vi "BRig_RT_start_v1,05__PortC.vi"() -> ()   [LabVIEW 2014]
uses:
  myRIO_BRig_RT__Case_Exp_stateList.ctl
  myRIO_BRig_RT__Case_NonExp_stateList.ctl
  <vilib>/WebDAVClient/Advanced/SessionHandle.ctl
  <vilib>/Platform/TimedLoop/XDataNode/timing_clust.ctl
  <vilib>/Platform/TimedLoop/XDataNode/nitl_modes.ctl
  <vilib>/Platform/TimedLoop/XDataNode/wakeup.ctl
  <vilib>/myRIO/Common/Instrument Driver Framework/myRIO v1.0/UART/vis/myRIO v1.0 Close UART.vi
  <vilib>/FPGAPlugInAG/myRIO-1900/niLvFpga_Open_myRIO-1900.vi
  <vilib>/rvi/interface/common/dynamic/niFpgaDynamicAddResources.vi
  <vilib>/Utility/error.llb/Error Cluster From Error Code.vi
  <vilib>/rvi/errors/niLvFpgaAdjustHostInterfaceError.vi
  <vilib>/Utility/file.llb/Read From Spreadsheet File (I64).vi
  <vilib>/Utility/file.llb/Write To Spreadsheet File (DBL).vi
  <vilib>/FPGAPlugInAG/Dynamic/niLvFpga_Close_Dynamic.vi
  <vilib>/myRIO/Common/Instrument Driver Framework/Utilities/vis/FPGA Ref Manager.vi
  <vilib>/myRIO/Common/Instrument Driver Framework/myRIO v1.0/myRIO v1.0 Reset FPGA.vi
  <vilib>/myRIO/Common/Instrument Driver Framework/myRIO v1.0/IRQ/vis/myRIO v1.0 IRQ Info FGV.vi
  <vilib>/myRIO/Common/Instrument Driver Framework/myRIO v1.0/IRQ/vis/myRIO v1.0 Timer IRQ Info FGV.vi
  <vilib>/myRIO/Common/Instrument Driver Framework/myRIO v1.0/IRQ/vis/myRIO v1.0 ISR Agent.vi
  <vilib>/rvi/interface/nirviOpenFPGA/nirviOpenFPGA.xnode
  BRig_FPGA_v3,91__PortC__build.lvbitx
  BRig_FPGA_v3,91__PortC.vi
  <vilib>/rvi/interface/nirviReadWriteControl/nirviReadWriteControl.xnode
  <vilib>/Platform/TimedLoop/XDataNode/XDataNode.xnode
  <vilib>/rvi/interface/nirviCloseFPGA/nirviCloseFPGA.xnode
  <vilib>/Platform/TimedLoop/XDataNode/XDNodeRunTimeDep.lvlib
  <vilib>/rvi/interface/Simulation/niFpgaSimulationCallBeginRW.vi
  <vilib>/myRIO/Instrument Drivers/Utilities/Utilities.lvlib
  NiFpgaLv.dll
  <vilib>/WebDAVClient/NI_WebDAV.lvlib
panel:
  out "FreeReward_c_R":u16
  out "FreeReward_c_L":u16
  in  "Laser2_LED":bool
  in  "Laser1_LED":bool
  in  "lick_Rising(F)_or_Falling(T)":bool
  out "T_ExpRun_min":dbl
  out "stop_TimedLoop":bool
  out "BTPR_avg_R":dbl
  out "T2R_avg_R":dbl
  out "BTPR_avg_L":dbl
  out "T2R_avg_L":dbl
  out "BTPR_block":u16
  out "T2R_block":u16
  in  "comm_WebDAV_connect":bool
  in  "I_sendData":bool
  in  "comm_TCP_connect":bool
  out "nRewards_total":u16 caption="# Rewards in Current Block"
  out "BUR_target":u16 caption="Target Trials Per Block"
  in  "input_Threshold_reset":bool
  out "nTrial":u16
  out "allReward_R":bool
  out "allReward_L":bool
  out "Threshold":bool
  out "tLoop":dbl format="%#_2g"
  out "L_Power_l2":dbl
  out "comm_TCP":bool
  in  "get_countPerMS":bool
  out "SolenoidReward":bool
  out "L_Power_l1":dbl caption="LaserPower"
  in  "Recording":bool
  out "FPGA_count2ms":dbl=159.0
  out "error out":errorcluster
  out "cSpout":enum16{"Left", "Right"}(ring) caption="Left or Right Spout"
  out "A4":u32 caption="LickCounter_Right"
  out "A2":u32 caption="LickCounter_Left"
  out "nRewards_Right":u16 caption="# Rewards Total (Right)"
  out "nRewards_Left":u16 caption="# Rewards Total (Left)"
  out "nRewards_cur":u16 caption="# Rewards in Current Block"
  out "TpB_target":u16 caption="Target Trials Per Block"
  out "cState_NonExp":T1 caption="WarmUp State"
  out "iBlock":u16 caption="Current Block"
  out "cState":T2 caption="Experimental State"
  out "iTrial":u16 caption="Current Trial"
  in  "Data Set Prefix":string="Exp1_TM2"
  out "comm_WebDAV":bool
  in  "Host Password":string="sabalab"
  in  "Host UserName":string="Test2"
  in  "STOP_abort":bool caption="Stop LabView\n(Stops myRio and FPGA)"
  in  "STOP_endBlock":bool caption="Stop Experiment\n@ End of Block"
  in  "STOP_endTrial":bool caption="Stop Experiment\n@ End of Trial"
  in  "START":bool caption="Start Experiment"
  # "Experimental Run"
  # "Recording Rig"
  # "FPGA Conversion\n[counts per ms]"
  # "RealTime Cycle\nShould be <5ms"
  # "STOP experiment at"
  # "Exp Run Time"
  # "Reset"
  # "min"
  # "Communication with Host"
  # "Test AnalogInput Plotting"
  # "Lick Counter"
  # "Give Water?\n(Reward)"
  # "Experimental State"
  # "Left/Right"
  # "AI0               AI1"
  # "Left           Right"
  # "Direction\n(NonSpecific Licking)"
  # "Block Target"
  # "# Blocks"
  # "L          R"
  # "# Trials"
  # "# Rewards"
  # "Bad Trials\nPost Reward"
  # "Trials 2 Reward"
  # "Block"
  # "# Trials"
  # "# Rewards"
  # "Current\nBlock"
  # "WarmUp State"
  # "avg L"
  # "Total"
  # "# Rewards"
  # "# Trials"
  # "avg R"
  # "Laser Power [V]"
  # "Left           Right"
  # "FreeRewards"
  # "Laser1"
  # "Laser2"
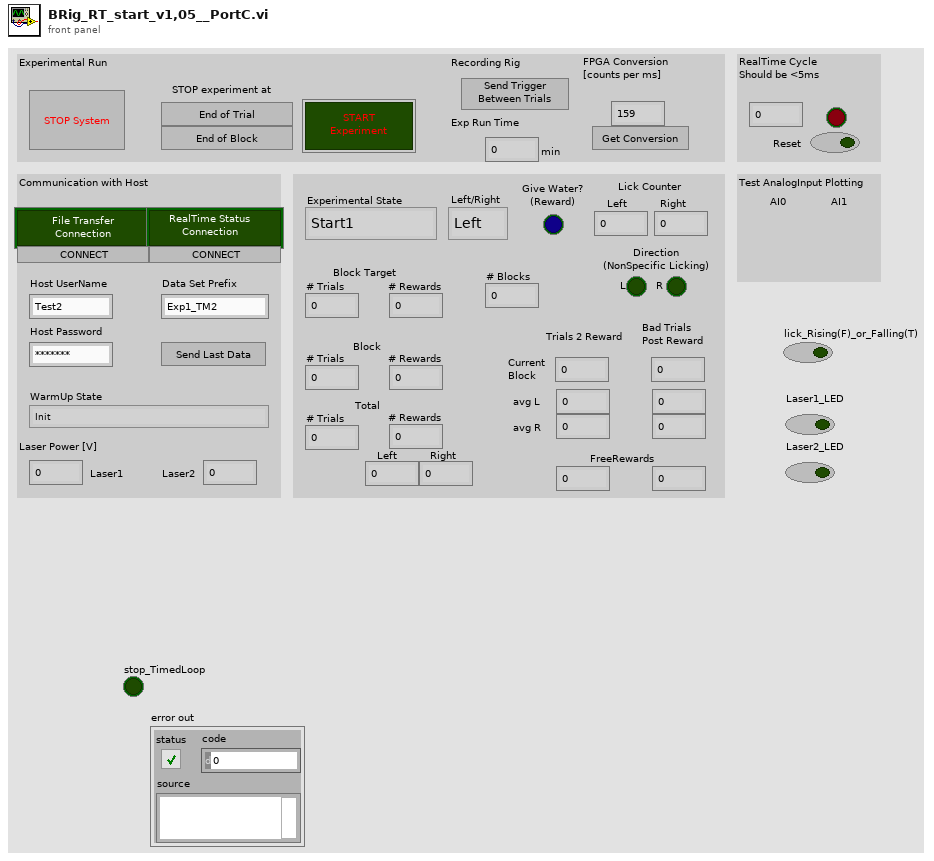
[diagram p1: front panel]
types:
  T1 = typedef "myRIO_BRig_RT__Case_NonExp_stateList.ctl" = enum16{"Init", "UploadSettings_pre", "UploadSettings_Read_dataExp", "UploadSettings_dataExp_1", "UploadSettings_dataExp_2", "UploadSettings_Read_dataLC", "UploadSettings_dataLC_1", "UploadSettings_dataLC_2", "UploadSettings_dataLC_3", "UploadSettings_dataLC_4", "UploadSettings_Read_dataMTrig", "UploadSettings_dataMTrig_1", "UploadSettings_post", "Idle_pre", "IdleEmpty", "IdleEmpty2", "IdleEmpty3", "IdleEmpty4", "Idle", "Idle_2", "Idle_3", "Idle_4", "Idle_5", "Idle_6", "Idle_post", "Cue_pre__pre", "Cue_pre", "Cue", "Cue_LED", "Cue_post", "RewardCalibration_pre", "RewardCalibration", "DispenseWater_pre__pre", "DispenseWater_pre", "DispenseWater", "DispenseWater_post", "TestConnection", "SendData", "Get_FPGA_count_per_ms", "End", "commTCP_connect"}
  T2 = typedef "myRIO_BRig_RT__Case_Exp_stateList.ctl" = enum16{"Start1", "Start2", "Start3", "saveSettings1", "saveSettings2", "saveSettings3", "saveSettings4", "saveSettings_LC_ENL_l1", "saveSettings_LC_ENL_l2", "saveSettings_LC_Cue_l1", "saveSettings_LC_Cue_l2", "saveSettings6_LC_l1_Other", "SaveSettings6_LC_l2_Other", "setSettings_Audio", "setSettings_Laser", "initBlock_pre", "initBlock", "initBlock2", "initBlock_post", "initTrial_pre", "initTrial", "initTrial2", "initTrial3", "initTrial4", "initTrial_LC_ENL1", "initTrial_LC_Cue1", "initTrial_LC_Cue1_2", "initTrial_LC_Sel", "initTrial_post", "ENL1_pre", "ENL1", "ENL1_post", "ENL1Penalty_pre", "ENL1Penalty", "ENL2_pre", "ENL2", "ENL2Penalty_pre", "ENL2Penalty", "Cue1_pre", "Cue1", "Cue1_post", "Cue1Penalty_pre", "Cue1Penalty", "Cue2_pre", "Cue2", "Cue2Penalty_pre", "Cue2Penalty", "Selection_pre", "Selection", "Select_post", "SelectReward_pre", "SelectReward", "SelectRewardPost_pre", "SelectRewardPost", "SelectWrong_pre", "SelectWrong", "SelectWrong_post", "SelectTimeout_pre", "SelectTimeout", "SelectTimeout_post", "endTrial_pre", "endTrial1", "endTrial2", "endTrial3", "endTrial_post", "endBlock_pre", "endBlock", "endBlock_post", "endExp", "commConnect", "commUpload_pre", "commUpload_dataBlock", "commUpload_dataCurrent", "commUpload_dataExp", "commUpload_dataLC", "commUpload_dataTrial", "commUpload_post", "saveData_pre", "saveData_dataBlock", "saveData_dataCurrent", "saveData_dataExp", "saveData_dataLC", "saveData_dataTrial", "saveData_post", "empty_endBlock1", "empty_endBlock2", "empty_endTrial1", "empty_endTrial2", "empty_endTrial3", "empty_endTrial4", "empty_endTrial5", "dummyState", "dummyState_endBlock", "FreeReward_pre", "FreeReward", "FreeRewardPost_pre", "FreeRewardPost"}
  T3 = enum8{"Enabled", "Disabled", "Disabled and Grayed Out"}
  T4 = typedef "NI_WebDAV.lvlib/SessionHandle.ctl" = refnum<k1>
  T5 = typedef "XDNodeRunTimeDep.lvlib/timing_clust.ctl" = cluster{"Expected End [f-1]":u64, "Actual End [f-1]":u64, "Finished Late? [f-1]":bool, "Expected End [i-1]":u64, "Actual End [i-1]":u64, "Finished Late? [i-1]":bool, "Expected Start [i]":u64, "Actual Start [i]":u64, "Expected Start [f]":u64, "Actual Start [f]":u64, "Source Name":string, "Structure Name":string, "Period":i64, "Deadline":i64, "Offset":i64, "Start":i64, "Priority":i32, "Timeout":i32, "Mode":T6, "Wakeup Reason":T7, "Error":errorcluster, "Source Type":string, "Secondary Source Type":string, "Global End Time":u64, "Global Start Time":u64, "Frame Duration":u64, "Iteration Duration":u64, "Assigned CPU":i32, "I/O Scan Engine Mode":u32}
  T6 = typedef "XDNodeRunTimeDep.lvlib/nitl_modes.ctl" = enum32{"No Change", "Process missed periods, maintain original phase", "Discard missed periods, maintain original phase", "Process missed periods, ignore original phase", "Discard missed periods, ignore original phase"}
  T7 = typedef "XDNodeRunTimeDep.lvlib/wakeup.ctl" = enum32{"Normal", "Aborted", "Asynchronous wakeup", "Timing source error", "Timed loop error", "Timeout"}
  T8 = cluster{"read mode":enum16{"polling", "blocking"}, "write mode":enum16{"polling", "blocking"}}
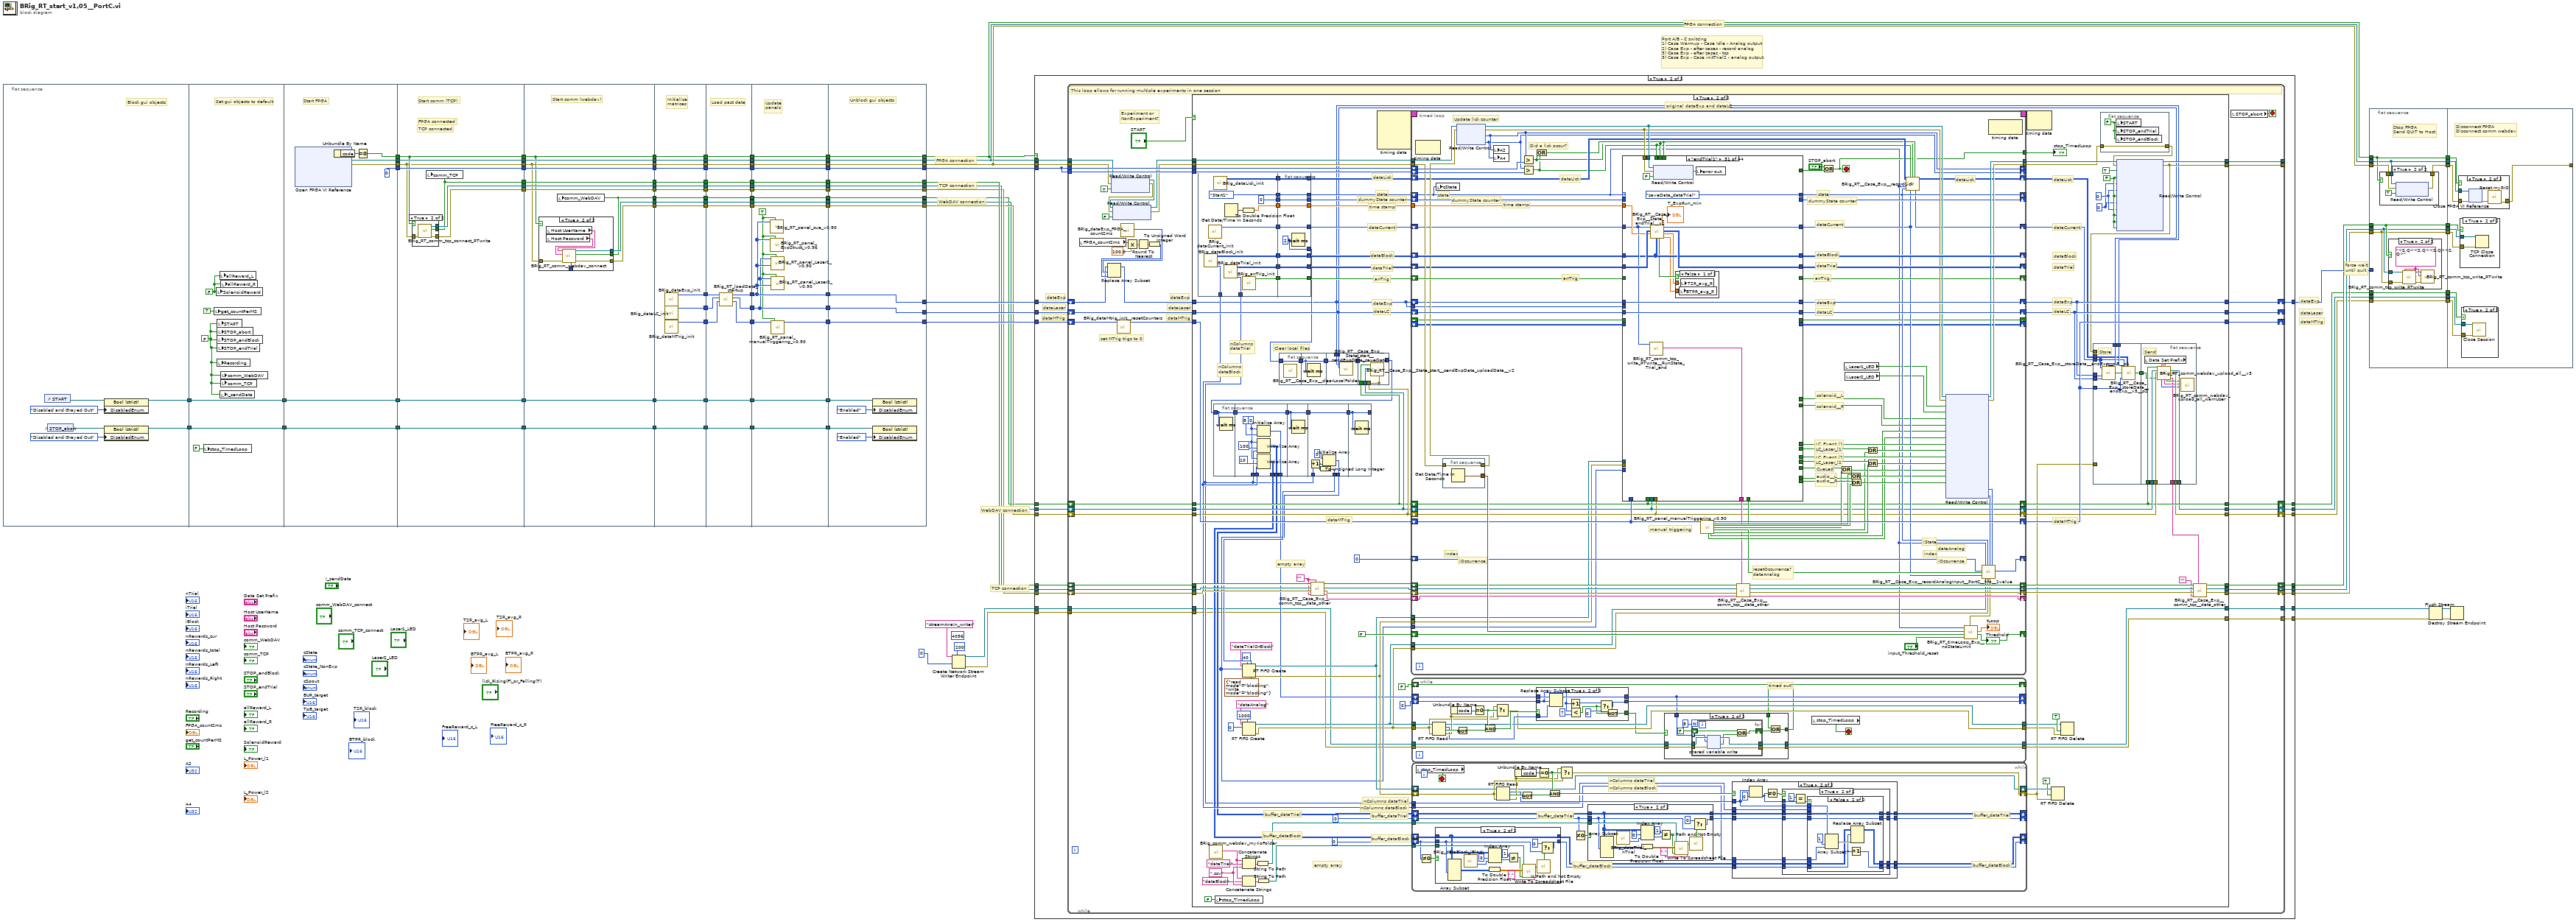
[diagram p0: block diagram]
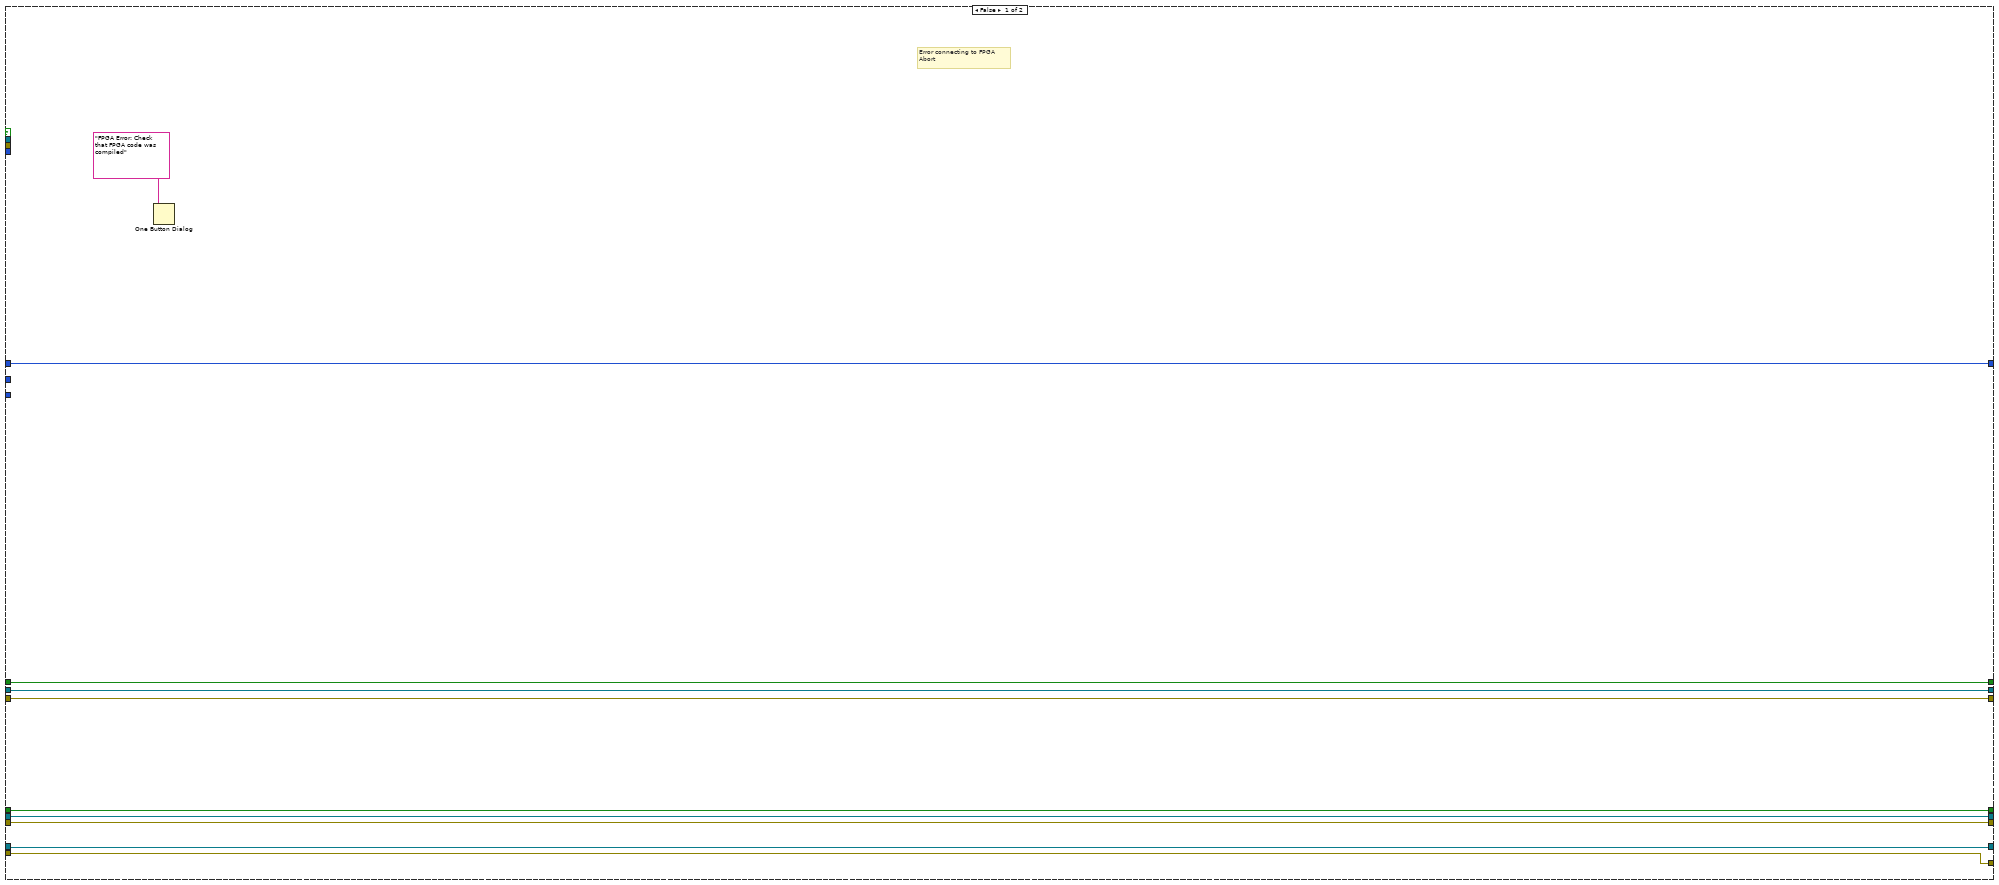
[diagram p2: hidden frame]
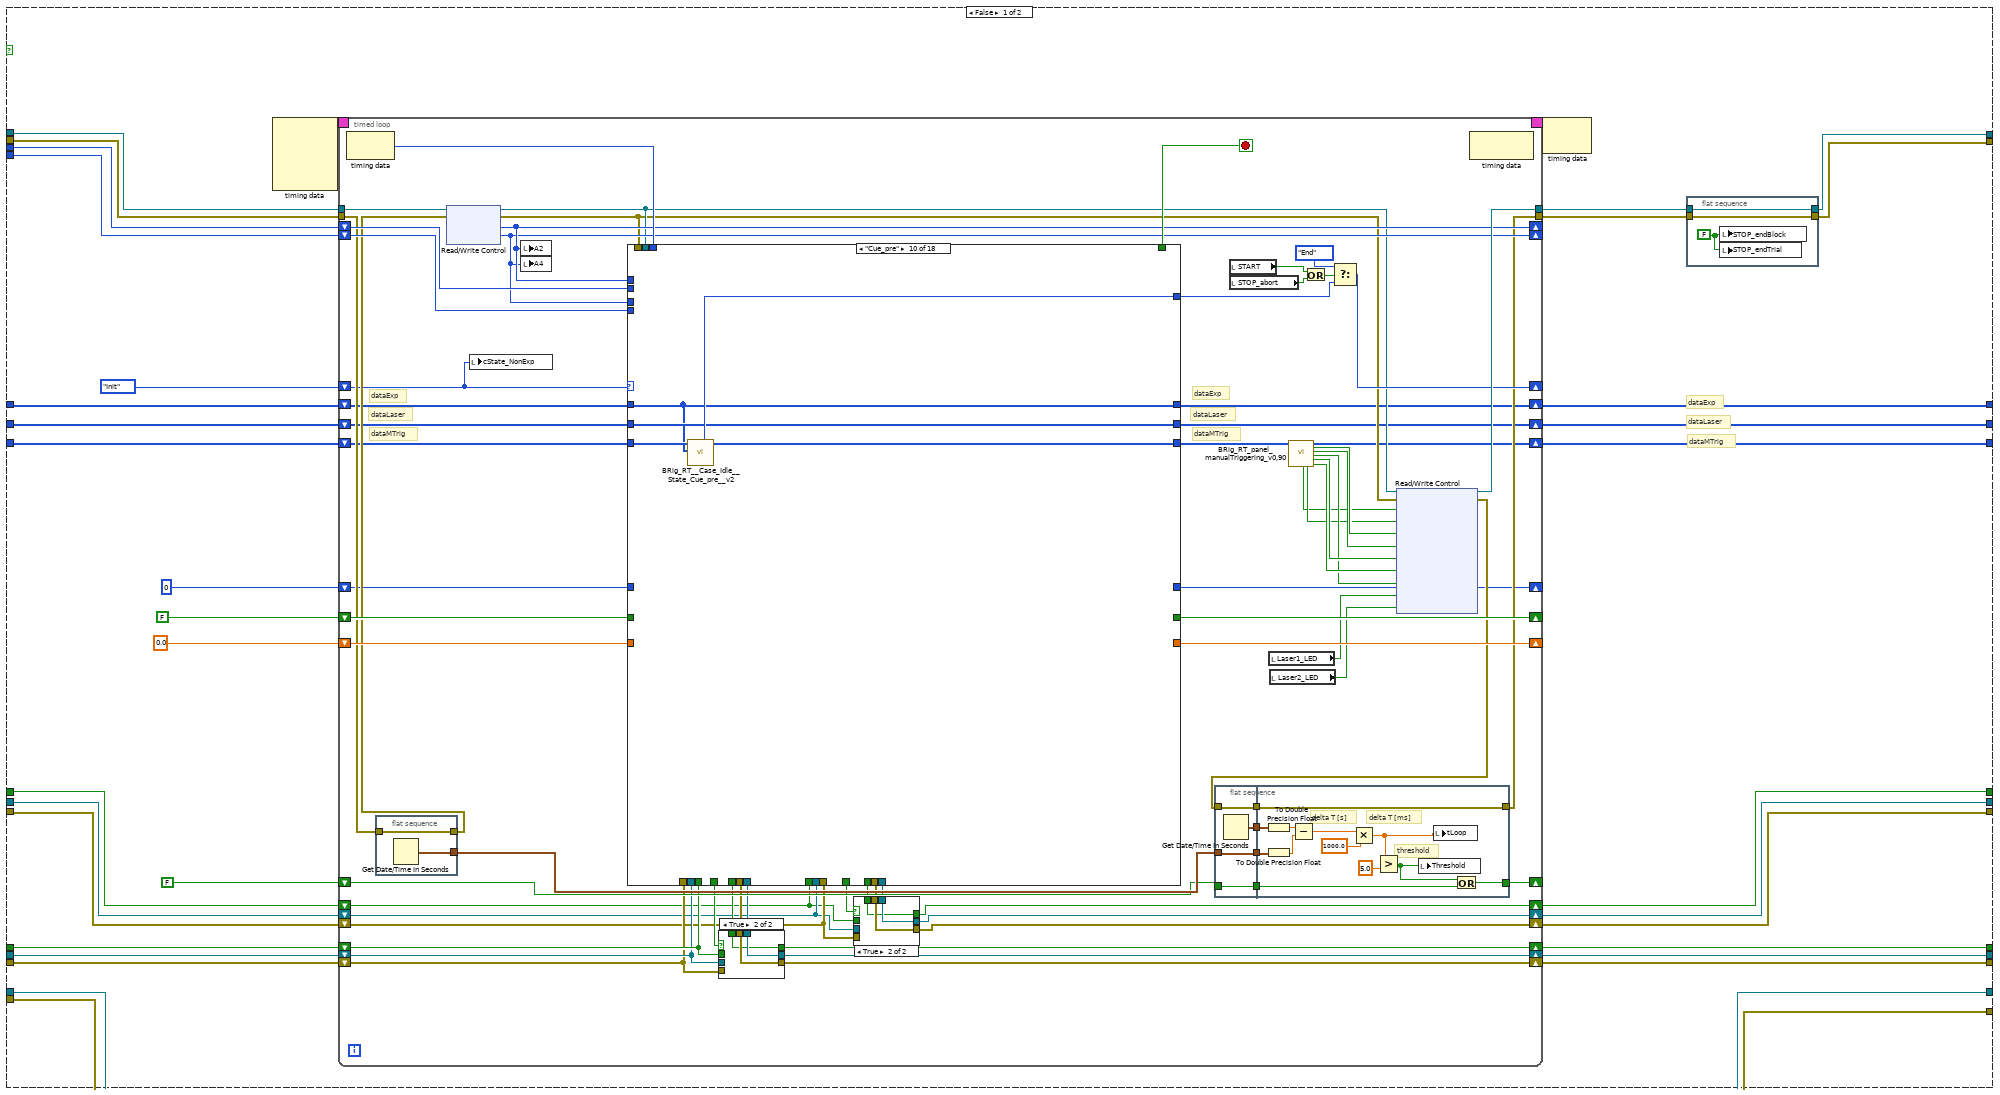
[diagram p3: hidden frame]
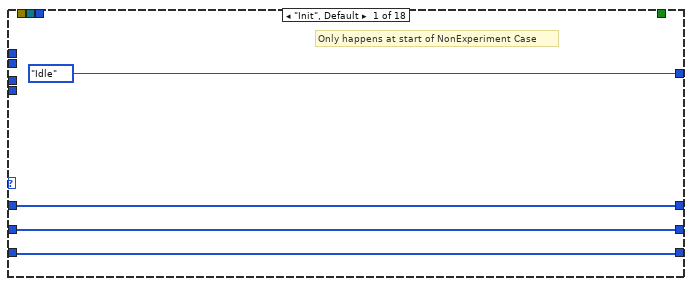
[diagram p6: hidden frame]
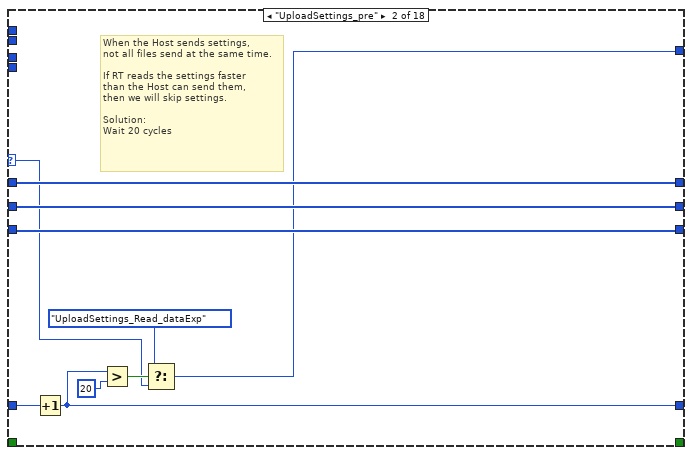
[diagram p7: hidden frame]
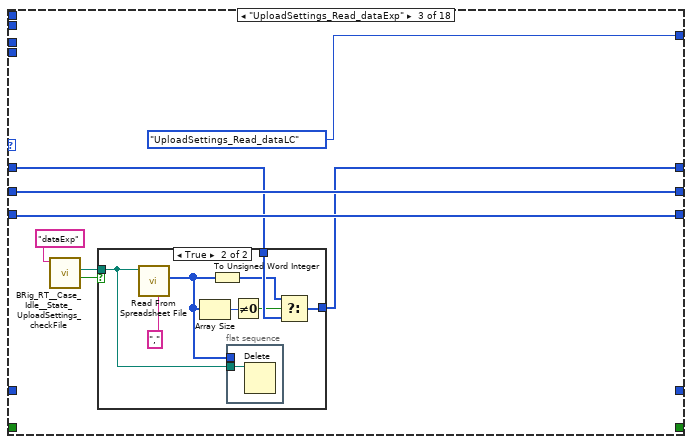
[diagram p8: hidden frame]
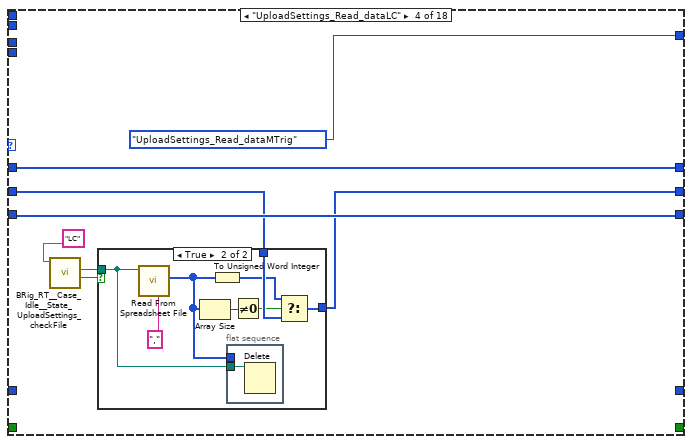
[diagram p10: hidden frame]
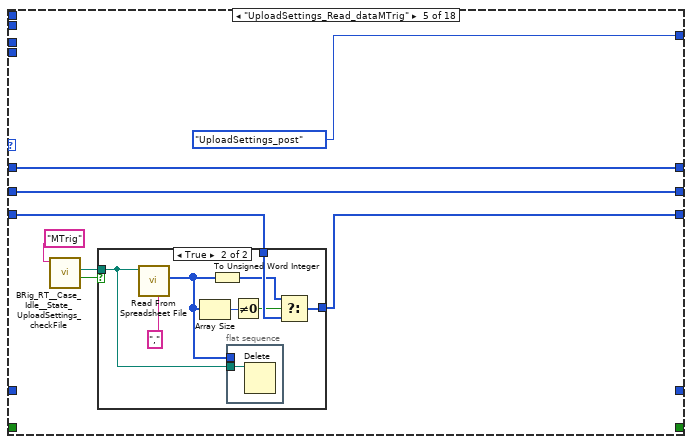
[diagram p12: hidden frame]
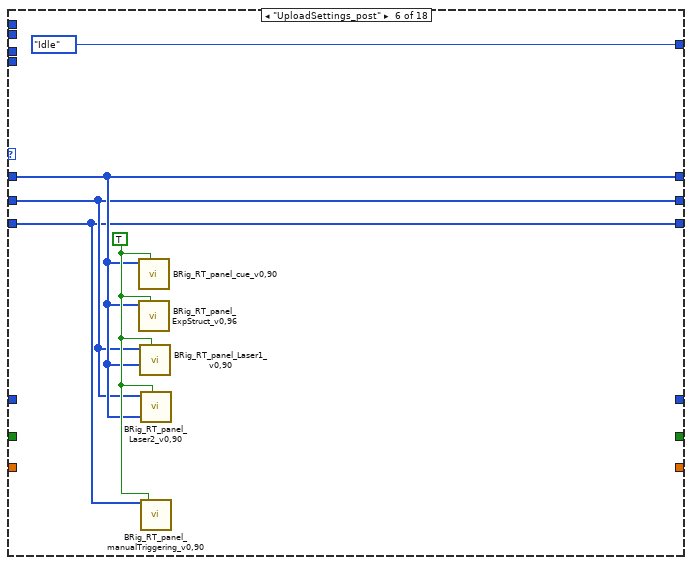
[diagram p14: hidden frame]
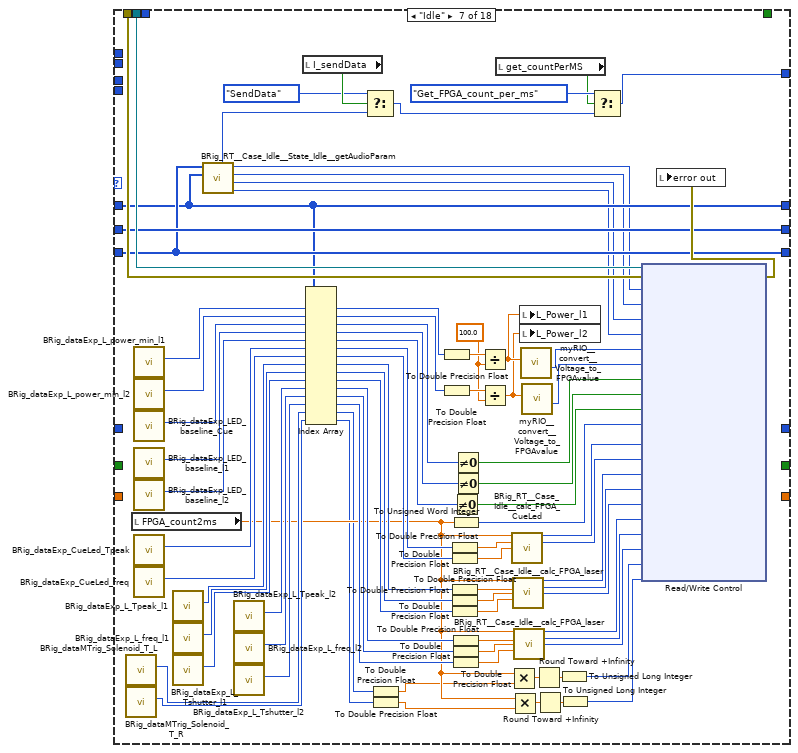
[diagram p15: hidden frame]
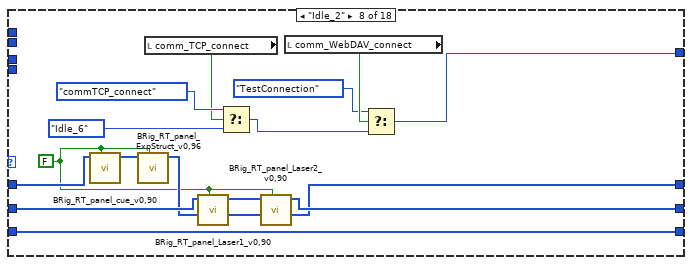
[diagram p16: hidden frame]
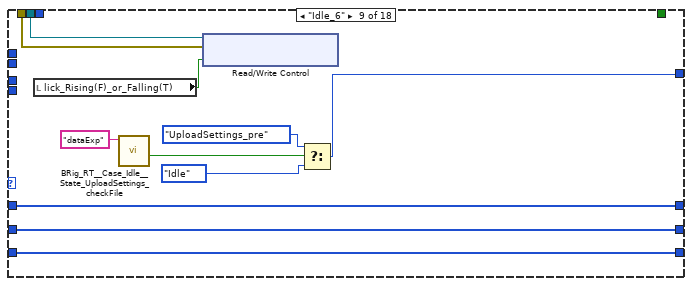
[diagram p17: hidden frame]
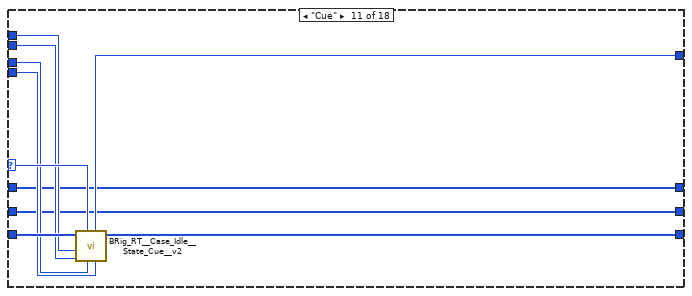
[diagram p18: hidden frame]
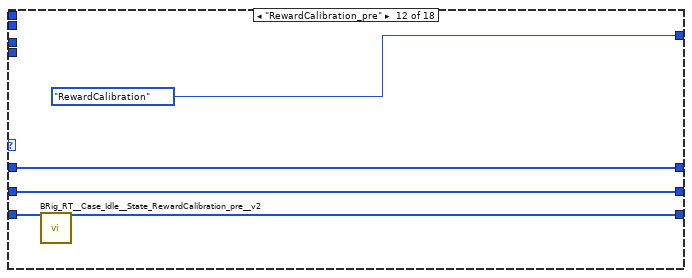
[diagram p19: hidden frame]
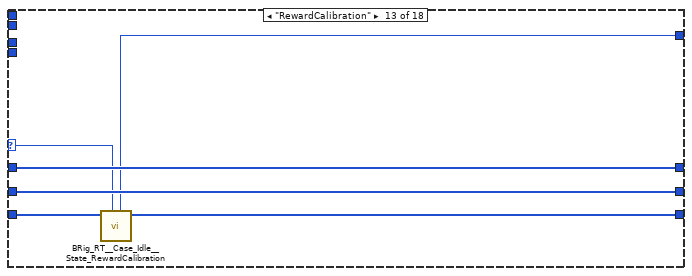
[diagram p20: hidden frame]
diagram:
  (unwired) 4096 ("reader buffer size")
  # "WebDAV connection"
  # "TCP connection"
  # "WebDAV connection"
  # "TCP connection"
  # "FPGA connection"
  # "FPGA connection"
  # "Port A/B - C switcing\n1) Case Warmup - Case Idle - Analog output\n2) Case Exp - after cases - record analog\n3) Case Exp - after cases - tcp\n3) Case Exp - Case initTrial2 - analog output"
  # "force wait\nuntil quit"
  # "dataLaser"
  # "dataExp"
  # "dataMTrig"
  n1 = flat-sequence {
    tunnel: [w116] -> w99
    tunnel: [w115] -> w95
    tunnel: [w125] -> w100
    tunnel: w99 -> [w125]
    tunnel: [w124] -> w96
    tunnel: w95 -> [w124]
    tunnel: [w131] -> w113
    tunnel: [w133] -> w112
    tunnel: [u32 0] -> w111
    tunnel: [w129] -> w110
    tunnel: [w128] -> w101
    tunnel: w100 -> [w128]
    tunnel: [w127] -> w97
    tunnel: w96 -> [w127]
    tunnel: w113 -> [w139]
    tunnel: w112 -> [w142]
    tunnel: w111 -> [w141]
    tunnel: w110 -> [w140]
    tunnel: [w139] -> w109
    tunnel: [w142] -> w108
    tunnel: [w141] -> w107
    tunnel: [w140] -> w106
    tunnel: [w134] -> w105
    tunnel: [w138] -> w104
    tunnel: [w137] -> w103
    tunnel: [w136] -> w102
    tunnel: w101 -> [w136]
    tunnel: [w135] -> w98
    tunnel: w97 -> [w135]
    tunnel: w109 -> [w153]
    tunnel: w108 -> [w161]
    tunnel: w107 -> [w160]
    tunnel: w106 -> [w154]
    tunnel: w105 -> [w159]
    tunnel: w104 -> [w158]
    tunnel: w103 -> [w157]
    tunnel: [w153] -> w66
    tunnel: [w161] -> w65
    tunnel: [w160] -> w64
    tunnel: [w154] -> w63
    tunnel: [w159] -> w62
    tunnel: [w158] -> w61
    tunnel: [w157] -> w60
    tunnel: [w156] -> w59
    tunnel: w102 -> [w156]
    tunnel: [w155] -> w58
    tunnel: w98 -> [w155]
    tunnel: [w152] -> w57
    tunnel: [w150] -> w56
    tunnel: [w151] -> w55
    tunnel: w66 -> [w186]
    tunnel: [w186] -> w54
    tunnel: w65 -> [w185]
    tunnel: [w185] -> w53
    tunnel: w64 -> [w184]
    tunnel: [w184] -> w52
    tunnel: w63 -> [w183]
    tunnel: [w183] -> w51
    tunnel: w62 -> [w182]
    tunnel: [w182] -> w50
    tunnel: w61 -> [w181]
    tunnel: [w181] -> w49
    tunnel: w60 -> [w180]
    tunnel: [w180] -> w48
    tunnel: w59 -> [w179]
    tunnel: [w179] -> w47
    tunnel: w58 -> [w178]
    tunnel: [w178] -> w46
    tunnel: w57 -> [w177]
    tunnel: [w177] -> w45
    tunnel: w56 -> [w176]
    tunnel: [w176] -> w44
    tunnel: w55 -> [w175]
    tunnel: [w175] -> w43
    tunnel: [w174] -> w42
    tunnel: [w173] -> w41
    tunnel: [w172] -> w40
    tunnel: w54 -> [w204]
    tunnel: [w204] -> w39
    tunnel: w53 -> [w203]
    tunnel: [w203] -> w37
    tunnel: w52 -> [w202]
    tunnel: [w202] -> w35
    tunnel: w51 -> [w201]
    tunnel: [w201] -> w33
    tunnel: w50 -> [w200]
    tunnel: [w200] -> w31
    tunnel: w49 -> [w199]
    tunnel: [w199] -> w29
    tunnel: w48 -> [w198]
    tunnel: [w198] -> w27
    tunnel: w47 -> [w197]
    tunnel: [w197] -> w25
    tunnel: w46 -> [w196]
    tunnel: [w196] -> w23
    tunnel: w45 -> [w195]
    tunnel: [w195] -> w21
    tunnel: w44 -> [w194]
    tunnel: [w194] -> w19
    tunnel: w43 -> [w193]
    tunnel: [w193] -> w17
    tunnel: w42 -> [w188]
    tunnel: [w187] -> w15
    tunnel: w41 -> [w190]
    tunnel: [w189] -> w13
    tunnel: w40 -> [w192]
    tunnel: [w191] -> w12
    tunnel: w39 -> [w221]
    tunnel: [w221] -> w38
    tunnel: w37 -> [w220]
    tunnel: [w220] -> w36
    tunnel: w35 -> [w219]
    tunnel: [w219] -> w34
    tunnel: w33 -> [w218]
    tunnel: [w218] -> w32
    tunnel: w31 -> [w217]
    tunnel: [w217] -> w30
    tunnel: w29 -> [w216]
    tunnel: [w216] -> w28
    tunnel: w27 -> [w215]
    tunnel: [w215] -> w26
    tunnel: w25 -> [w214]
    tunnel: [w214] -> w24
    tunnel: w23 -> [w213]
    tunnel: [w213] -> w22
    tunnel: w21 -> [w212]
    tunnel: [w212] -> w20
    tunnel: w19 -> [w211]
    tunnel: [w211] -> w18
    tunnel: w17 -> [w210]
    tunnel: [w210] -> w16
    tunnel: w15 -> [w207]
    tunnel: [w206] -> w14
    tunnel: w13 -> [w208]
    tunnel: w12 -> [w209]
    tunnel: [w209] -> w11
    tunnel: [w208] -> w10
    tunnel: [w228] -> w76
    tunnel: [w229] -> w77
    tunnel: [w230] -> w78
    tunnel: [w235] -> w82
    tunnel: [w236] -> w114
    tunnel: [w237] -> w89
    tunnel: [w238] -> w88
    tunnel: w38 -> [w238]
    tunnel: w36 -> [w237]
    tunnel: w34 -> [w236]
    tunnel: w32 -> [w235]
    tunnel: w30 -> [w230]
    tunnel: w28 -> [w229]
    tunnel: w26 -> [w228]
    tunnel: w24 -> [w232]
    tunnel: w22 -> [w231]
    tunnel: w20 -> [w226]
    tunnel: w18 -> [w227]
    tunnel: w16 -> [w225]
    tunnel: [w227] -> w70
    tunnel: [w226] -> w71
    tunnel: [w225] -> w72
    tunnel: [w222] -> w85
    tunnel: [w223] -> w84
    tunnel: [w224] -> w83
    tunnel: w14 -> [w224]
    tunnel: w11 -> [w222]
    tunnel: w10 -> [w223]
    frame #0 {
      # "Block gui objects"
      n2 = control-ref of="START"() -> (w120:refnum<vi>)
      n3 = control-ref of="STOP_abort"() -> (w117:refnum<vi>)
      n4 = property class="Bool (strict)"(reference=w120, "DisabledEnum"=T3."Disabled and Grayed Out" ("Disabled")) -> (reference out=w116:refnum<vi>)  [unwired: 1 in, 1 out]
      n5 = property class="Bool (strict)"(reference=w117, "DisabledEnum"=T3."Disabled and Grayed Out" ("Disabled")) -> (reference out=w115:refnum<vi>)  [unwired: 1 in, 1 out]
    }
    frame #1 {
      w122 = FALSE ("SolenoidReward")
      w123 = FALSE
      # "Set gui objects to default"
      n6 = local write "stop_TimedLoop"(FALSE ("stop_TimedLoop")) -> ()
      n7 = local write "get_countPerMS"(TRUE ("get_countPerMS")) -> ()
      n8 = local write "SolenoidReward"(w122) -> ()
      n9 = local write "START"(w123) -> ()
      n10 = local write "STOP_abort"(w123) -> ()
      n11 = local write "STOP_endBlock"(w123) -> ()
      n12 = local write "STOP_endTrial"(w123) -> ()
      n13 = local write "Recording"(w123) -> ()
      n14 = local write "allReward_L"(w122) -> ()
      n15 = local write "I_sendData"(w123) -> ()
      n16 = local write "comm_WebDAV"(w123) -> ()
      n17 = local write "comm_TCP"(w123) -> ()
      n18 = local write "allReward_R"(w122) -> ()
    }
    frame #2 {
      # "Start FPGA"
      n19 = xnode "Open FPGA VI Reference"() -> ("FPGA VI Reference Out"=w133:refnum<k20>, "error out"=w131:errorcluster)  [unwired: 2 in]
      n20 = Unbundle By Name(w131) -> ("code"=w130:i32)
      n21 = Equal To 0?(x=w130) -> (x = 0?=w129:bool)
    }
    frame #3 {
      # "TCP connected"
      # "Start comm (TCP)"
      # "FPGA connected"
      n22 = case shown="True" w140 {
        selector: w140 -> [w143 _]
        tunnel: w139 -> [w145 w149]
        tunnel: [refnum<k5> refnum ("output_hTCP") w148] -> w138
        tunnel: [w143 w147] -> w134
        tunnel: [w145 w146] -> w137
        frame False {
        }
        frame True {
          n23 = call "BRig_RT_comm_tcp_connect_RTwrite.vi"("input_error"=w149) -> ("output_error"=w146:errorcluster, "output_connected"=w147:bool, "output_hTCP"=w148:refnum<k5>)  [unwired: 8 in]
        }
      }
      n24 = local write "comm_TCP"(w134) -> ()
    }
    frame #4 {
      # "Start comm (webdav)"
      n25 = case shown="True" w154 {
        selector: w154 -> [w163 _]
        tunnel: [w162 w169] -> w152
        tunnel: [w163 w168] -> w150
        tunnel: w153 -> [w164 w167]
        tunnel: [w164 w166] -> w151
        tunnel: [_ w165] -> _
        frame False {
          w162 = T4 refnum items=["Session NI_WebDAV"] ("output_hSession")
        }
        frame True {
          n26 = local read "Host UserName"() -> (w170:string)
          n27 = local read "Host Password"() -> (w171:string)
          n28 = call "BRig_RT_comm_webdav_connect.vi"("input_error"=w167, "input_password"=w171, "input_username"=w170) -> ("output_error"=w166:errorcluster, "output_Iconnected"=w168:bool, "output_hSession"=w169:T4, "output_code"=w165:u8)  [unwired: 5 in]
        }
      }
      n29 = local write "comm_WebDAV"(w150) -> ()
    }
    frame #5 {
      # "Initialize\nmatrices"
      n30 = call "BRig_dataExp_init.vi"() -> ("output_dataExp"=w172:u16[])  [unwired: 11 in]
      n31 = call "BRig_dataLC_init.vi"() -> ("output_dataLC"=w173:u16[])  [unwired: 11 in]
      n32 = call "BRig_dataMTrig_init.vi"() -> ("output_dataMTrig"=w174:u16[])  [unwired: 5 in]
    }
    frame #6 {
      # "Load past data"
      n33 = call "BRig_RT_loadData_startup.vi"("input_dataMTrig"=w188, "input_dataLC"=w190, "input_dataExp"=w192) -> ("output_dataMTrig"=w187:u16[], "output_dataLC"=w189:u16[], "output_dataExp"=w191:u16[])  [unwired: 6 in]
    }
    frame #7 {
      w205 = TRUE ("input_setValues")
      # "Update\npanels"
      n34 = call "BRig_RT_panel_cue_v0,90.vi"("input_setValues"=w205, "input_dataExp"=w209) -> ()  [unwired: 9 in, 1 out]
      n35 = call "BRig_RT_panel_ExpStruct_v0,96.vi"("input_setValues"=w205, "input_dataExp"=w209) -> ()  [unwired: 9 in, 1 out]
      n36 = call "BRig_RT_panel_Laser1_v0,90.vi"("input_setValues"=w205, "input_dataExp"=w209, "input_dataLC"=w208) -> ()  [unwired: 7 in, 2 out]
      n37 = call "BRig_RT_panel_Laser2_v0,90.vi"("input_setValues"=w205, "input_dataExp"=w209, "input_dataLC"=w208) -> ()  [unwired: 7 in, 2 out]
      n38 = call "BRig_RT_panel_manualTriggering_v0,90.vi"("input_dataMTrig"=w207, "input_setValues"=w205) -> ("output_dataMTrig"=w206:u16[])  [unwired: 10 in, 7 out]
    }
    frame #8 {
      # "Unblock gui objects"
      n39 = property class="Bool (strict)"(reference=w232, "DisabledEnum"=T3."Enabled" ("Disabled")) -> ()  [unwired: 1 in, 2 out]
      n40 = property class="Bool (strict)"(reference=w231, "DisabledEnum"=T3."Enabled" ("Disabled")) -> ()  [unwired: 1 in, 2 out]
    }
  }
  n41 = Create Network Stream Writer Endpoint(7:200 ("reader buffer size"), 9:u16 0 ("element"), 11:"streamAnaIn_writer" ("reader name")) -> (0:w2:errorcluster, 3:w3:refnum<k21>)  [unwired: 4 in]
  n42 = case shown="True" w82 {
    tunnel: w114 -> [_ w271]
    tunnel: w89 -> [_ w270]
    tunnel: w88 -> [_ w269]
    tunnel: [w248 w268] -> w86
    tunnel: w85 -> [w248 w267]
    tunnel: w84 -> [_ w266]
    tunnel: w83 -> [_ w265]
    tunnel: w78 -> [w247 w264]
    tunnel: w77 -> [w246 w263]
    tunnel: w76 -> [w245 w262]
    tunnel: [w247 w261] -> w75
    tunnel: [w246 w260] -> w74
    tunnel: [w245 w259] -> w73
    tunnel: w72 -> [w244 w258]
    tunnel: w71 -> [w243 w257]
    tunnel: w70 -> [w242 w256]
    tunnel: [w244 w255] -> w69
    tunnel: [w243 w254] -> w68
    tunnel: [w242 w253] -> w67
    tunnel: [w241 w252] -> w7
    tunnel: [w240 w251] -> w6
    tunnel: w3 -> [w241 w250]
    tunnel: w2 -> [w240 w249]
    frame False {
      # "Error connecting to FPGA\nAbort"
      n43 = One Button Dialog(message="FPGA Error: Check that FPGA code was compiled") -> ()  [unwired: 1 in, 1 out]
    }
    frame True {
      # "dataExp"
      # "dataLaser"
      # "dataMTrig"
      n44 = while {
        tunnel: w270 -> [w305]
        tunnel: w269 -> [w310]
        tunnel: w271 -> [w313]
        tunnel: w271 -> [w312]
        tunnel: [w303] -> _
        tunnel: [w302] -> _
        shift-right: [w301] -> _
        shift-left: w265 -> [w297]
        shift-right: [w299] -> _
        shift-left: w266 -> [w300]
        shift-right: [w298] -> w268
        shift-left: w267 -> [w277]
        shift-right: [w292] -> w261
        shift-left: w264 -> [w295]
        shift-right: [w291] -> w260
        shift-left: w263 -> [w294]
        shift-right: [w290] -> w259
        shift-left: w262 -> [w293]
        shift-right: [w286] -> w255
        shift-left: w258 -> [w289]
        shift-right: [w285] -> w254
        shift-left: w257 -> [w288]
        shift-right: [w284] -> w253
        shift-left: w256 -> [w287]
        tunnel: [w275] -> w252
        tunnel: [w274] -> w251
        tunnel: w250 -> [w273]
        tunnel: w249 -> [w272]
        stop <- w311 stop-if-true
        # "set MTrig trigs to 0"
        # "dataExp"
        # "dataLaser"
        # "dataMTrig"
        # "Experiment or\nNonExperiment?"
        # "This loop allows for running multiple experiments in one session"
        n45 = local read "FPGA_count2ms"() -> (w281:dbl)
        n46 = xnode "Read/Write Control"("FPGA VI Reference In"=w305, "error in"=w310, "Counts_Reset"=TRUE) -> ("FPGA VI Reference Out"=w307:refnum<k20>, "error out"=w308:errorcluster)
        n47 = xnode "Read/Write Control"("FPGA VI Reference In"=w307, "error in"=w308, "Counts_Reset"=FALSE) -> ("FPGA VI Reference Out"=w304:refnum<k20>, "error out"=w306:errorcluster)
        n48 = call "BRig_dataMtrig_init__resetCounters.vi"("input_dataMTrig"=w297) -> ("output_dataMTrig"=w296:u16[])  [unwired: 10 in]
        n49 = call "BRig_dataExp_FPGA_count2ms.vi"() -> ("output_FPGA_count2ms"=w282:i32)  [unwired: 11 in]
        n50 = Multiply(x=w281, y=100.0) -> (x*y=w279:dbl)
        n51 = Round To Nearest(number=w279) -> (nearest integer value=w278:dbl)
        n52 = To Unsigned Word Integer(number=w278) -> (unsigned 16bit integer=w283:u16)
        n53 = Replace Array Subset(array=w277, new element=w283, index=w282) -> (w276:u16[])
        n54 = case shown="True" "START" {
          tunnel: w313 -> [w347 w909]
          tunnel: w312 -> [w346 w908]
          tunnel: w306 -> [w344 w897]
          tunnel: w304 -> [w345 w898]
          tunnel: [w342 w906] -> w303
          tunnel: [w340 w875] -> w302
          tunnel: w296 -> [w336 w895]
          tunnel: [w335 w881] -> w301
          tunnel: w300 -> [w334 w845]
          tunnel: w276 -> [w333 w796]
          tunnel: [w332 w880] -> w299
          tunnel: [w331 w879] -> w298
          tunnel: w295 -> [w330 w889]
          tunnel: w294 -> [w329 w888]
          tunnel: w293 -> [w328 w887]
          tunnel: [w327 w864] -> w292
          tunnel: [w326 w863] -> w291
          tunnel: [w325 w862] -> w290
          tunnel: w289 -> [w324 w844]
          tunnel: w288 -> [w323 w843]
          tunnel: w287 -> [w322 w842]
          tunnel: [w321 w871] -> w286
          tunnel: [w320 w870] -> w285
          tunnel: [w319 w872] -> w284
          tunnel: w273 -> [w317 w801]
          tunnel: w272 -> [w316 w800]
          tunnel: [w317 w799] -> w275
          tunnel: [w316 w798] -> w274
          frame False {
            # "dataExp"
            # "dataLaser"
            # "dataMTrig"
            n55 = node-c288() -> (w350:T5)  [unwired: 4 in]
            n56 = timed-loop {
              timing: w350 -> [_]
              timing-out: [_] -> w349
              shift-right: [w414] -> _
              shift-left: myRIO_BRig_RT__Case_NonExp_stateList."Init" ("Enum") -> [w383]
              shift-right: [w412] -> _
              shift-left: w347 -> [w413]
              shift-right: [w410] -> _
              shift-left: w346 -> [w411]
              tunnel: [w420] -> w343
              tunnel: [w396] -> w341
              tunnel: w344 -> [w403]
              tunnel: w345 -> [w421]
              shift-right: [w406] -> _
              shift-left: FALSE -> [w407]
              shift-right: [w404] -> _
              shift-left: 0.0 -> [w405]
              shift-right: [w393] -> _
              shift-left: FALSE -> [w394]
              shift-right: [w392] -> w335
              shift-left: w336 -> [w384]
              shift-right: [w378] -> w331
              shift-left: w333 -> [w381]
              shift-right: [w379] -> w332
              shift-left: w334 -> [w380]
              shift-right: [w377] -> w327
              shift-left: w330 -> [w373]
              shift-right: [w376] -> w326
              shift-left: w329 -> [w372]
              shift-right: [w375] -> w325
              shift-left: w328 -> [w371]
              shift-right: [w361] -> w321
              shift-left: w324 -> [w367]
              shift-right: [w362] -> w320
              shift-left: w323 -> [w366]
              shift-right: [w363] -> w319
              shift-left: w322 -> [w365]
              shift-right: [w356] -> _
              shift-left: u16 0 ("y") -> [w357]
              stop <- w423 stop-if-true
              # "dataExp"
              # "dataLaser"
              # "dataExp"
              # "dataLaser"
              # "dataMTrig"
              # "dataMTrig"
              n57 = node-c288() -> (w422:i64)  [unwired: 1 in]
              n58 = flat-sequence {
                tunnel: w403 -> [w452]
                tunnel: [w453] -> w395
                tunnel: [w452] -> w402
                frame #0 {
                  n59 = Get Date/Time In Seconds() -> (seconds since 1Jan1904=w453:timestamp)
                }
              }
              n60 = xnode "Read/Write Control"("FPGA VI Reference In"=w421, "error in"=w402) -> ("FPGA VI Reference Out"=w409:refnum<k20>, "error out"=w408:errorcluster, "A2_LickL"=w412:u32, "A4_LickR"=w410:u32)
              n61 = local write "cState_NonExp"(w383) -> ()
              n62 = local write "A2"(w412) -> ()
              n63 = local write "A4"(w410) -> ()
              n64 = case shown="\"Cue_pre\"" w383 {
                selector: w383 -> [_ w460 _ _ _ _ _ _ _ _ w651 _ w659 _ _ w702 w745 w751]
                tunnel: [myRIO_BRig_RT__Case_NonExp_stateList."Idle" ("Enum") w461 myRIO_BRig_RT__Case_NonExp_stateList."UploadSettings_Read_dataLC" ("t") myRIO_BRig_RT__Case_NonExp_stateList."UploadSettings_Read_dataMTrig" ("t") myRIO_BRig_RT__Case_NonExp_stateList."UploadSettings_post" ("t") myRIO_BRig_RT__Case_NonExp_stateList."Idle" ("t") w542 w610 w634 w640 w649 myRIO_BRig_RT__Case_NonExp_stateList."RewardCalibration" ("Enum") w658 myRIO_BRig_RT__Case_NonExp_stateList."Idle" ("Enum") myRIO_BRig_RT__Case_NonExp_stateList."Idle" ("Enum") w701 w745 w752] -> w415
                tunnel: [w456 w467 w475 w493 w507 w522 w554 w626 w632 w641 w650 w653 w660 w674 w686 w711 w743 w760] -> w382
                tunnel: [_ _ _ _ _ _ _ _ _ _ _ _ _ _ _ _ TRUE _] -> w423
                tunnel: w384 -> [w456 w467 w475 w493 w504 w522 w554 w626 w632 w642 w652 w654 w661 w674 w686 w711 w743 w760]
                tunnel: w422 -> [_ _ _ _ _ _ _ _ _ _ _ _ _ _ _ _ _ _]
                tunnel: w413 -> [_ _ _ _ _ _ _ _ _ _ w647 _ _ _ _ _ _ _]
                tunnel: w412 -> [_ _ _ _ _ _ _ _ _ _ w648 _ _ _ _ _ _ _]
                tunnel: w411 -> [_ _ _ _ _ _ _ _ _ _ w645 _ _ _ _ _ _ _]
                tunnel: w410 -> [_ _ _ _ _ _ _ _ _ _ w646 _ _ _ _ _ _ _]
                tunnel: w409 -> [_ _ _ _ _ _ w609 _ w629 _ _ _ _ _ _ w706 _ _]
                tunnel: w408 -> [_ _ _ _ _ _ w608 _ w628 _ _ _ _ _ _ w705 _ _]
                tunnel: w407 -> [_ _ _ _ _ _ _ _ _ _ _ _ _ _ _ w710 _ _]
                tunnel: [_ _ _ _ _ _ _ _ _ _ _ _ _ _ _ TRUE _ _] -> w406
                tunnel: w405 -> [_ _ _ _ _ _ _ _ _ _ _ _ _ _ _ w708 _ _]
                tunnel: [_ _ _ _ _ _ _ _ _ _ _ _ _ _ _ w707 _ _] -> w404
                tunnel: w381 -> [w454 w465 w470 w492 w511 w524 w553 w624 w630 w638 w643 w656 w662 w671 w683 w698 w741 w758]
                tunnel: w380 -> [w455 w466 w474 w486 w508 w523 w555 w623 w631 w639 w644 w655 w663 w672 w684 w699 w742 w759]
                tunnel: [w455 w466 w474 w489 w508 w523 w555 w619 w631 w639 w644 w655 w663 w672 w684 w699 w742 w759] -> w379
                tunnel: [w454 w465 w469 w492 w511 w524 w553 w616 w630 w638 w643 w656 w662 w671 w683 w698 w741 w758] -> w378
                tunnel: [_ _ _ _ _ _ _ _ _ _ _ _ _ _ _ _ _ TRUE] -> w374
                tunnel: w373 -> [_ _ _ _ _ _ _ _ _ _ _ _ _ _ w677 _ _ w757]
                tunnel: w372 -> [_ _ _ _ _ _ _ _ _ _ _ _ _ _ w679 _ _ w753]
                tunnel: w371 -> [_ _ _ _ _ _ _ _ _ _ _ _ _ _ w678 _ _ w756]
                tunnel: [_ _ _ _ _ _ _ _ _ _ _ _ _ _ _ _ _ w755] -> w370
                tunnel: [_ _ _ _ _ _ _ _ _ _ _ _ _ _ _ _ _ w754] -> w369
                tunnel: [_ _ _ _ _ _ _ _ _ _ _ _ _ _ _ _ _ w746] -> w368
                tunnel: w365 -> [_ _ _ _ _ _ _ _ _ _ _ _ _ _ w676 _ _ _]
                tunnel: w366 -> [_ _ _ _ _ _ _ _ _ _ _ _ _ _ w682 _ _ _]
                tunnel: w367 -> [_ _ _ _ _ _ _ _ _ _ _ _ _ w664 w681 _ _ _]
                tunnel: [_ _ _ _ _ _ _ _ _ _ _ _ _ TRUE _ _ _ _] -> w364
                tunnel: [_ _ _ _ _ _ _ _ _ _ _ _ _ w666 _ _ _ _] -> w360
                tunnel: [_ _ _ _ _ _ _ _ _ _ _ _ _ w664 _ _ _ _] -> w359
                tunnel: [_ _ _ _ _ _ _ _ _ _ _ _ _ w665 _ _ _ _] -> w358
                tunnel: w357 -> [_ w459 _ _ _ _ _ _ _ _ _ _ _ _ _ _ _ _]
                tunnel: [_ w458 _ _ _ _ _ _ _ _ _ _ _ _ _ _ _ _] -> w356
                frame "Init", Default {
                  # "Only happens at start of NonExperiment Case"
                }
                frame "UploadSettings_pre" {
                  # "When the Host sends settings,\nnot all files send at the same time.\n\nIf RT reads the settings faster\nthan the Host can send them,\nthen we will skip settings.\n\nSolution:\nWait 20 cycles"
                  n65 = Increment(x=w459) -> (x+1=w458:u16)
                  n66 = Greater?(x=w458, y=u16 20) -> (0:w463:bool)
                  n67 = Select(t=myRIO_BRig_RT__Case_NonExp_stateList."UploadSettings_Read_dataExp", s=w463, f=w460) -> (s? t:f=w461:T1)
                }
                frame "UploadSettings_Read_dataExp" {
                  n68 = call "BRig_RT__Case_Idle__State_UploadSettings_checkFile.vi"("input_dataName"="dataExp") -> ("output_Iexist"=w472:bool, "output_dataPath"=w471:path)  [unwired: 9 in]
                  n69 = case shown="True" w472 {
                    tunnel: w471 -> [_ w478]
                    tunnel: w470 -> [w476 w482]
                    tunnel: [w476 w480] -> w469
                    frame False {
                    }
                    frame True {
                      n70 = call-poly <vilib>:"Read From Spreadsheet File.vi"("delimiter (\\t)"="," ("delimiter (\\t)"), "file path (dialog if empty)"=w478) -> ("first row"=w477:i64[])  [unwired: 5 in, 4 out]
                      n71 = Array Size(array=w477) -> (size(s)=w483:i32)
                      n72 = To Unsigned Word Integer(number=w477) -> (unsigned 16bit integer=w481:u16[])
                      n73 = flat-sequence {
                        tunnel: w478 -> [w485]
                        tunnel: w477 -> [_]
                        frame #0 {
                          n74 = Delete(path (use dialog)=w485) -> ()  [unwired: 4 in, 3 out]
                        }
                      }
                      n75 = Not Equal To 0?(x=w483) -> (x != 0?=w479:bool)
                      n76 = Select(t=w481, s=w479, f=w482) -> (s? t:f=w480:u16[])
                    }
                  }
                }
                frame "UploadSettings_Read_dataLC" {
                  n77 = call "BRig_RT__Case_Idle__State_UploadSettings_checkFile.vi"("input_dataName"="LC") -> ("output_Iexist"=w487:bool, "output_dataPath"=w488:path)  [unwired: 9 in]
                  n78 = case shown="True" w487 {
                    tunnel: w488 -> [_ w496]
                    tunnel: w486 -> [w494 w500]
                    tunnel: [w494 w498] -> w489
                    frame False {
                    }
                    frame True {
                      n79 = call-poly <vilib>:"Read From Spreadsheet File.vi"("delimiter (\\t)"="," ("delimiter (\\t)"), "file path (dialog if empty)"=w496) -> ("first row"=w495:i64[])  [unwired: 5 in, 4 out]
                      n80 = Array Size(array=w495) -> (size(s)=w501:i32)
                      n81 = To Unsigned Word Integer(number=w495) -> (unsigned 16bit integer=w499:u16[])
                      n82 = flat-sequence {
                        tunnel: w496 -> [w503]
                        tunnel: w495 -> [_]
                        frame #0 {
                          n83 = Delete(path (use dialog)=w503) -> ()  [unwired: 4 in, 3 out]
                        }
                      }
                      n84 = Not Equal To 0?(x=w501) -> (x != 0?=w497:bool)
                      n85 = Select(t=w499, s=w497, f=w500) -> (s? t:f=w498:u16[])
                    }
                  }
                }
                frame "UploadSettings_Read_dataMTrig" {
                  n86 = call "BRig_RT__Case_Idle__State_UploadSettings_checkFile.vi"("input_dataName"="MTrig") -> ("output_Iexist"=w505:bool, "output_dataPath"=w506:path)  [unwired: 9 in]
                  n87 = case shown="True" w505 {
                    tunnel: w506 -> [_ w514]
                    tunnel: w504 -> [w512 w518]
                    tunnel: [w512 w516] -> w507
                    frame False {
                    }
                    frame True {
                      n88 = call-poly <vilib>:"Read From Spreadsheet File.vi"("delimiter (\\t)"="," ("delimiter (\\t)"), "file path (dialog if empty)"=w514) -> ("first row"=w513:i64[])  [unwired: 5 in, 4 out]
                      n89 = Array Size(array=w513) -> (size(s)=w519:i32)
                      n90 = To Unsigned Word Integer(number=w513) -> (unsigned 16bit integer=w517:u16[])
                      n91 = flat-sequence {
                        tunnel: w514 -> [w521]
                        tunnel: w513 -> [_]
                        frame #0 {
                          n92 = Delete(path (use dialog)=w521) -> ()  [unwired: 4 in, 3 out]
                        }
                      }
                      n93 = Not Equal To 0?(x=w519) -> (x != 0?=w515:bool)
                      n94 = Select(t=w517, s=w515, f=w518) -> (s? t:f=w516:u16[])
                    }
                  }
                }
                frame "UploadSettings_post" {
                  w525 = TRUE ("input_setValues")
                  n95 = call "BRig_RT_panel_cue_v0,90.vi"("input_setValues"=w525, "input_dataExp"=w524) -> ()  [unwired: 9 in, 1 out]
                  n96 = call "BRig_RT_panel_ExpStruct_v0,96.vi"("input_setValues"=w525, "input_dataExp"=w524) -> ()  [unwired: 9 in, 1 out]
                  n97 = call "BRig_RT_panel_Laser1_v0,90.vi"("input_setValues"=w525, "input_dataExp"=w524, "input_dataLC"=w523) -> ()  [unwired: 7 in, 2 out]
                  n98 = call "BRig_RT_panel_Laser2_v0,90.vi"("input_setValues"=w525, "input_dataExp"=w524, "input_dataLC"=w523) -> ()  [unwired: 7 in, 2 out]
                  n99 = call "BRig_RT_panel_manualTriggering_v0,90.vi"("input_dataMTrig"=w522, "input_setValues"=w525) -> ()  [unwired: 10 in, 8 out]
                }
                frame "Idle" {
                  w599 = 100.0 ("y")
                  n100 = call "BRig_dataMTrig_Solenoid_T_L.vi"() -> ("output_Solenoid_T_L"=w537:i32)  [unwired: 11 in]
                  n101 = call "BRig_dataMTrig_Solenoid_T_R.vi"() -> ("output_Solenoid_T_R"=w536:i32)  [unwired: 11 in]
                  n102 = local read "FPGA_count2ms"() -> (w535:dbl)
                  n103 = call "BRig_dataExp_L_power_min_l1.vi"() -> ("output_L_power_min_l1"=w604:i32)  [unwired: 11 in]
                  n104 = call "BRig_dataExp_L_power_min_l2.vi"() -> ("output_L_power_min_l2"=w603:i32)  [unwired: 11 in]
                  n105 = call "BRig_dataExp_LED_baseline_Cue.vi"() -> ("output_LED_baseline_Cue"=w597:i32)  [unwired: 11 in]
                  n106 = call "BRig_dataExp_LED_baseline_l1.vi"() -> ("output_LED_baseline_l1"=w596:i32)  [unwired: 11 in]
                  n107 = call "BRig_dataExp_LED_baseline_l2.vi"() -> ("output_LED_baseline_l2"=w595:i32)  [unwired: 11 in]
                  n108 = call "BRig_dataExp_CueLed_Tpeak.vi"() -> ("output_CueLed_Tpeak"=w587:i32)  [unwired: 11 in]
                  n109 = call "BRig_dataExp_CueLed_freq.vi"() -> ("output_CueLed_Freq"=w586:i32)  [unwired: 11 in]
                  n110 = call "BRig_dataExp_L_Tpeak_l1.vi"() -> ("output_L_Tpeak_l1"=w579:i32)  [unwired: 11 in]
                  n111 = call "BRig_dataExp_L_freq_l1.vi"() -> ("output_L_freq_l1"=w578:i32)  [unwired: 11 in]
                  n112 = call "BRig_dataExp_L_Tshutter_l1.vi"() -> ("output_L_Tshutter_l1"=w577:i32)  [unwired: 11 in]
                  n113 = call "BRig_RT__Case_Idle__State_Idle__getAudioParam.vi"("input_dataExp"=w553, "input_dataMTrig"=w554) -> ("output_Audio_freq_R"=w549:u8, "output_Audio_amp_R"=w550:u16, "output_Audio_freq_L"=w551:u8, "output_Audio_amp_L"=w552:u16, "output_state"=w548:T1)  [unwired: 5 in]
                  n114 = call "BRig_dataExp_L_Tpeak_l2.vi"() -> ("output_L_Tpeak_l2"=w561:i32)  [unwired: 11 in]
                  n115 = call "BRig_dataExp_L_freq_l2.vi"() -> ("output_L_freq_l2"=w560:i32)  [unwired: 11 in]
                  n116 = call "BRig_dataExp_L_Tshutter_l2.vi"() -> ("output_L_Tshutter_l2"=w559:i32)  [unwired: 11 in]
                  n117 = local read "I_sendData"() -> (w547:bool)
                  n118 = Index Array(array=w553, index #1=w604, index #2=w603, index #3=w597, index #4=w596, index #5=w595, index #6=w587, index #7=w586, index #8=w579, index #9=w578, index #10=w577, index #11=w561, index #12=w560, index #13=w559, index #14=w537, index #15=w536) -> (element #1=w602:u16, element #2=w598:u16, element #3=w594:u16, element #4=w593:u16, element #5=w592:u16, element #6=w583:u16, element #7=w582:u16, element #8=w576:u16, element #9=w575:u16, element #10=w574:u16, element #11=w564:u16, element #12=w563:u16, element #13=w562:u16, element #14=w534:u16, element #15=w533:u16)
                  n119 = Select(t=myRIO_BRig_RT__Case_NonExp_stateList."SendData" ("Enum"), s=w547, f=w548) -> (s? t:f=w544:T1)
                  n120 = To Double Precision Float(number=w534) -> (double precision float=w532:dbl)
                  n121 = To Double Precision Float(number=w533) -> (double precision float=w531:dbl)
                  n122 = To Double Precision Float(number=w602) -> (double precision float=w601:dbl)
                  n123 = To Double Precision Float(number=w598) -> (double precision float=w600:dbl)
                  n124 = To Double Precision Float(number=w583) -> (double precision float=w585:dbl)
                  n125 = To Double Precision Float(number=w582) -> (double precision float=w584:dbl)
                  n126 = To Double Precision Float(number=w576) -> (double precision float=w573:dbl)
                  n127 = To Double Precision Float(number=w575) -> (double precision float=w572:dbl)
                  n128 = To Double Precision Float(number=w574) -> (double precision float=w571:dbl)
                  n129 = To Unsigned Word Integer(number=w535) -> (unsigned 16bit integer=w588:u16)
                  n130 = To Double Precision Float(number=w564) -> (double precision float=w565:dbl)
                  n131 = To Double Precision Float(number=w563) -> (double precision float=w566:dbl)
                  n132 = To Double Precision Float(number=w562) -> (double precision float=w567:dbl)
                  n133 = Not Equal To 0?(x=w592) -> (x != 0?=w589:bool)
                  n134 = Not Equal To 0?(x=w594) -> (x != 0?=w591:bool)
                  n135 = Not Equal To 0?(x=w593) -> (x != 0?=w590:bool)
                  n136 = Divide(x=w601, y=w599) -> (x/y=w528:dbl)
                  n137 = Divide(x=w600, y=w599) -> (x/y=w527:dbl)
                  n138 = local read "get_countPerMS"() -> (w543:bool)
                  n139 = Multiply(x=w535, y=w532) -> (x*y=w541:dbl)
                  n140 = Multiply(x=w535, y=w531) -> (x*y=w539:dbl)
                  n141 = call "BRig_RT__Case_Idle__calc_FPGA_CueLed.vi"("input_FPGA_ms2count"=w535, "input_Tpeak"=w585, "input_Freq"=w584) -> ("output_laser_Npeak"=w581:u32, "output_laser_Nvalley"=w580:u32)  [unwired: 11 in]
                  n142 = call "BRig_RT__Case_Idle__calc_FPGA_laser.vi"("input_FPGA_ms2count"=w535, "input_Tpeak"=w573, "input_Freq"=w572, "input_Tshutter"=w571) -> ("output_laser_Npeak"=w570:u32, "output_laser_Nvalley"=w569:u32, "output_laser_Nshutter"=w568:u32)  [unwired: 9 in]
                  n143 = call "BRig_RT__Case_Idle__calc_FPGA_laser.vi"("input_FPGA_ms2count"=w535, "input_Tpeak"=w565, "input_Freq"=w566, "input_Tshutter"=w567) -> ("output_laser_Npeak"=w558:u32, "output_laser_Nvalley"=w557:u32, "output_laser_Nshutter"=w556:u32)  [unwired: 9 in]
                  n144 = local write "L_Power_l1"(w528) -> ()
                  n145 = local write "L_Power_l2"(w527) -> ()
                  n146 = call "myRIO__convert__Voltage_to_FPGAvalue.vi"("input_voltage"=w528) -> ("output_PortC"=w605:i16)  [unwired: 9 in, 1 out]
                  n147 = call "myRIO__convert__Voltage_to_FPGAvalue.vi"("input_voltage"=w527) -> ("output_PortC"=w606:i16)  [unwired: 9 in, 1 out]
                  n148 = Round Toward +Infinity(x=w541) -> (ceil(x): smallest int >= x=w540:dbl)
                  n149 = Round Toward +Infinity(x=w539) -> (ceil(x): smallest int >= x=w538:dbl)
                  n150 = To Unsigned Long Integer(number=w540) -> (unsigned 32bit integer=w530:u32)
                  n151 = To Unsigned Long Integer(number=w538) -> (unsigned 32bit integer=w529:u32)
                  n152 = Select(t=myRIO_BRig_RT__Case_NonExp_stateList."Get_FPGA_count_per_ms" ("Enum"), s=w543, f=w544) -> (s? t:f=w542:T1)
                  n153 = xnode "Read/Write Control"("FPGA VI Reference In"=w609, "error in"=w608, "audioAmp_L"=w552, "audioFreq_L_kHz"=w551, "audioAmp_R"=w550, "audioFreq_R_kHz"=w549, "AnaOut_0"=w605, "AnaOut_1"=w606, "CueLed_Baseline"=w591, "L1Led_Baseline"=w590, "L2Led_Baseline"=w589, "k1__counter_per_ms"=w588, "CueLed_nPeak"=w581, "CueLed_nValley"=w580, "LC_nPeak_l1"=w570, "LC_nValley_l1"=w569, "LC_nShutter_l1"=w568, "LC_nPeak_l2"=w558, "LC_nValley_l2"=w557, "LC_nShutter_l2"=w556, "Solenoid_nTotal_L"=w530, "Solenoid_nTotal_R"=w529) -> ("error out"=w607:errorcluster)  [unwired: 1 out]
                  n154 = local write "error out"(w607) -> ()
                }
                frame "Idle_2" {
                  w615 = FALSE
                  n155 = call "BRig_RT_panel_cue_v0,90.vi"("input_setValues"=w615, "input_dataExp"=w624) -> ("output_dataExp"=w625:u16[])  [unwired: 9 in]
                  n156 = call "BRig_RT_panel_ExpStruct_v0,96.vi"("input_setValues"=w615, "input_dataExp"=w625) -> ("output_dataExp"=w618:u16[])  [unwired: 9 in]
                  n157 = local read "comm_TCP_connect"() -> (w614:bool)
                  n158 = call "BRig_RT_panel_Laser1_v0,90.vi"("input_setValues"=w615, "input_dataExp"=w618, "input_dataLC"=w623) -> ("output_dataExp"=w617:u16[], "output_dataLC"=w620:u16[])  [unwired: 7 in]
                  n159 = Select(t=myRIO_BRig_RT__Case_NonExp_stateList."commTCP_connect" ("Enum"), s=w614, f=myRIO_BRig_RT__Case_NonExp_stateList."Idle_6" ("Enum")) -> (s? t:f=w612:T1)
                  n160 = call "BRig_RT_panel_Laser2_v0,90.vi"("input_setValues"=w615, "input_dataExp"=w617, "input_dataLC"=w620) -> ("output_dataExp"=w616:u16[], "output_dataLC"=w619:u16[])  [unwired: 7 in]
                  n161 = local read "comm_WebDAV_connect"() -> (w613:bool)
                  n162 = Select(t=myRIO_BRig_RT__Case_NonExp_stateList."TestConnection" ("Enum"), s=w613, f=w612) -> (s? t:f=w610:T1)
                }
                frame "Idle_6" {
                  n163 = local read "lick_Rising(F)_or_Falling(T)"() -> (w627:bool)
                  n164 = call "BRig_RT__Case_Idle__State_UploadSettings_checkFile.vi"("input_dataName"="dataExp") -> ("output_Iexist"=w636:bool)  [unwired: 9 in, 1 out]
                  n165 = xnode "Read/Write Control"("FPGA VI Reference In"=w629, "error in"=w628, "Rising(F)_or_Falling(T)"=w627) -> ()  [unwired: 2 out]
                  n166 = Select(t=myRIO_BRig_RT__Case_NonExp_stateList."UploadSettings_pre" ("Enum"), s=w636, f=myRIO_BRig_RT__Case_NonExp_stateList."Idle") -> (s? t:f=w634:T1)
                }
                frame "Cue_pre" {
                  n167 = call "BRig_RT__Case_Idle__State_Cue_pre__v2.vi"("input_dataExp"=w638, "input_dataMTrig"=w642) -> ("output_dataMTrig"=w641:u16[], "output_state"=w640:T1)  [unwired: 8 in]
                }
                frame "Cue" {
                  n168 = call "BRig_RT__Case_Idle__State_Cue__v2.vi"("input_cLick_R_prev"=w645, "input_cLick_R"=w646, "input_state"=w651, "input_cLick_L_prev"=w647, "input_cLick_L"=w648, "input_dataMTrig"=w652) -> ("output_dataMTrig"=w650:u16[], "output_state"=w649:T1)  [unwired: 4 in]
                }
                frame "RewardCalibration_pre" {
                  n169 = call "BRig_RT__Case_Idle__State_RewardCalibration_pre__v2.vi"("input_dataMTrig"=w654) -> ("output_dataMTrig"=w653:u16[])  [unwired: 26 in]
                }
                frame "RewardCalibration" {
                  n170 = call "BRig_RT__Case_Idle__State_RewardCalibration.vi"("input_state"=w659, "input_dataMTrig"=w661) -> ("output_dataMtrig"=w660:u16[], "output_state"=w658:T1)  [unwired: 8 in]
                }
                frame "TestConnection" {
                  n171 = local read "Host Password"() -> (w667:string)
                  n172 = local read "Host UserName"() -> (w668:string)
                  n173 = call "BRig_RT_comm_webdav_connect.vi"("input_password"=w667, "input_username"=w668) -> ("output_Iconnected"=w666:bool, "output_hSession"=w665:T4)  [unwired: 6 in, 2 out]
                  n174 = local write "comm_WebDAV_connect"(FALSE ("comm_WebDAV_connect")) -> ()
                  n175 = local write "comm_WebDAV"(w666) -> ()
                }
                frame "SendData" {
                  n176 = And(x=w677, y=w676) -> (x .and. y?=w675:bool)
                  n177 = case shown="True" w675 {
                    tunnel: w676 -> [_ w693]
                    tunnel: w682 -> [_ w692]
                    tunnel: w681 -> [_ w691]
                    tunnel: w679 -> [_ w689]
                    tunnel: w678 -> [_ w688]
                    frame False {
                      n178 = One Button Dialog(message="Unable to send data:\n Missing one or more\n connections") -> ()  [unwired: 1 in, 1 out]
                    }
                    frame True {
                      n179 = local read "Data Set Prefix"() -> (w694:string)
                      n180 = call "BRig_RT_comm_webdav_upload_all.vi"("input_I_connected_webdav"=w693, "input_fileName_prefix"=w694, "input_hSession"=w692, "input_error"=w691) -> ("output_nFilenames"=w695:i32, "output_arrFilenames"=w696:string[], "output_uploaded"=w697:bool[], "output_strCmd"=w690:string)  [unwired: 6 in, 2 out]
                      n181 = call "BRig_RT_comm_tcp_write_RTwrite.vi"("input_error"=w688, "input_packet"=w690, "input_hTCP"=w689) -> ()  [unwired: 5 in, 4 out]
                      n182 = call "BRig_RT_comm_webdav_upload_all_warnUser.vi"("input_n"=w695, "input_arrFilenames"=w696, "input_arrUploaded"=w697) -> ()  [unwired: 9 in]
                    }
                  }
                  n183 = local write "I_sendData"(FALSE ("I_sendData")) -> ()
                }
                frame "Get_FPGA_count_per_ms" {
                  # "Used to automatically determine how many FPGA cycles in 1 ms"
                  n184 = case shown="True" w710 {
                    selector: w710 -> [w712 _]
                    tunnel: w708 -> [_ w725]
                    tunnel: [w716 w725] -> w707
                    tunnel: w706 -> [w715 w723]
                    tunnel: w705 -> [w714 w722]
                    tunnel: [w713 w720] -> w700
                    tunnel: [w712 w719] -> w704
                    frame False {
                      n185 = Get Date/Time In Seconds() -> (seconds since 1Jan1904=w717:timestamp)
                      n186 = To Double Precision Float(number=w717) -> (double precision float=w716:dbl)
                      n187 = xnode "Read/Write Control"("FPGA VI Reference In"=w715, "error in"=w714, "timeTrial_trig"=TRUE ("timeTrial")) -> ("error out"=w713:errorcluster)  [unwired: 1 out]
                      n188 = local write "get_countPerMS"(w712) -> ()
                    }
                    frame True {
                      w721 = 1.0
                      n189 = Get Date/Time In Seconds() -> (seconds since 1Jan1904=w726:timestamp)
                      n190 = To Double Precision Float(number=w726) -> (double precision float=w727:dbl)
                      n191 = Subtract(x=w727, y=w725) -> (x-y=w724:dbl)
                      n192 = Less Or Equal?(x=w721, y=w724) -> (x <= y?=w719:bool)
                      n193 = case shown="True" w719 {
                        tunnel: w723 -> [_ w740]
                        tunnel: w722 -> [w728 w739]
                        tunnel: w721 -> [_ w730]
                        tunnel: [w728 w729] -> w720
                        frame False {
                        }
                        frame True {
                          n194 = xnode "Read/Write Control"("FPGA VI Reference In"=w740, "error in"=w739) -> ("FPGA VI Reference Out"=w737:refnum<k20>, "error out"=w736:errorcluster, "timeTrial_count"=w731:u32)
                          n195 = Multiply(x=w730, y=1000.0) -> (x*y=w734:dbl)
                          n196 = To Double Precision Float(number=w731) -> (double precision float=w733:dbl)
                          n197 = Divide(x=w733, y=w734) -> (x/y=w735:dbl)
                          n198 = local write "FPGA_count2ms"(w735) -> ()
                          n199 = xnode "Read/Write Control"("FPGA VI Reference In"=w737, "error in"=w736, "timeTrial_trig"=FALSE ("timeTrial")) -> ("error out"=w729:errorcluster)  [unwired: 1 out]
                        }
                      }
                    }
                  }
                  n200 = Select(t=myRIO_BRig_RT__Case_NonExp_stateList."Idle" ("Enum"), s=w704, f=w702) -> (s? t:f=w701:T1)
                  n201 = local write "error out"(w700) -> ()
                }
                frame "End" {
                }
                frame "commTCP_connect" {
                  n202 = local read "comm_TCP_connect"() -> (w750:bool)
                  n203 = case shown="True" w757 {
                    tunnel: w756 -> [w767 w776]
                    tunnel: [w766 w772] -> w754
                    tunnel: [w765 w769] -> w746
                    tunnel: [w764 w770] -> w755
                    tunnel: w753 -> [_ w777]
                    frame False {
                      n204 = call "BRig_RT_comm_tcp_connect_RTwrite.vi"("input_error"=w767) -> ("output_error"=w764:errorcluster, "output_connected"=w765:bool, "output_hTCP"=w766:refnum<k5>)  [unwired: 8 in]
                    }
                    frame True {
                      n205 = call "BRig_RT_comm_tcp_write_RTwrite.vi"("input_error"=w776, "input_packet"="<test>", "input_hTCP"=w777) -> ("output_error"=w771:errorcluster, "output_I_NotDisconnected"=w768:bool, "output_I_write"=w774:bool, "output_hTCP"=w773:refnum<k5>)  [unwired: 5 in]
                      n206 = case shown="False" w774 {
                        selector: w774 -> [_ w788]
                        tunnel: w773 -> [w783 w790]
                        tunnel: [w778 w790] -> w772
                        tunnel: w771 -> [w782 w789]
                        tunnel: [w780 w789] -> w770
                        tunnel: [w779 w788] -> w769
                        tunnel: w768 -> [w784 _]
                        frame False {
                          n207 = case shown="True" w784 {
                            tunnel: w783 -> [_ w787]
                            tunnel: w782 -> [w785 w786]
                            tunnel: [w785 w786] -> w781
                            frame False {
                            }
                            frame True {
                              n208 = TCP Close Connection(connection ID=w787, error in (no error)=w786) -> ()  [unwired: 1 in, 2 out]
                            }
                          }
                          n209 = call "BRig_RT_comm_tcp_connect_RTwrite.vi"("input_error"=w781) -> ("output_error"=w780:errorcluster, "output_connected"=w779:bool, "output_hTCP"=w778:refnum<k5>)  [unwired: 8 in]
                        }
                        frame True {
                        }
                      }
                    }
                  }
                  n210 = Not(x=w750) -> (.not. x?=w749:bool)
                  n211 = Or(x=w749, y=w746) -> (x .or. y?=w748:bool)
                  n212 = case shown="True" w748 {
                    tunnel: [w761 myRIO_BRig_RT__Case_NonExp_stateList."Idle" ("Enum")] -> w752
                    tunnel: w751 -> [w761 _]
                    frame False {
                    }
                    frame True {
                      n213 = local write "comm_TCP_connect"(FALSE) -> ()
                    }
                  }
                  n214 = local write "comm_TCP"(w746) -> ()
                }
              }
              n215 = case shown="True" w374 {
                tunnel: [w432 w433] -> w377
                tunnel: [w431 w434] -> w376
                tunnel: [w430 w435] -> w375
                tunnel: w373 -> [w432 _]
                tunnel: w372 -> [w431 _]
                tunnel: w371 -> [w430 _]
                tunnel: w370 -> [_ w435]
                tunnel: w369 -> [_ w434]
                tunnel: w368 -> [_ w433]
                frame False {
                }
                frame True {
                }
              }
              n216 = case shown="True" w364 {
                tunnel: [w426 w427] -> w363
                tunnel: [w425 w428] -> w362
                tunnel: [w424 w429] -> w361
                tunnel: w365 -> [w426 _]
                tunnel: w366 -> [w425 _]
                tunnel: w367 -> [w424 _]
                tunnel: w359 -> [_ w429]
                tunnel: w358 -> [_ w428]
                tunnel: w360 -> [_ w427]
                frame False {
                }
                frame True {
                }
              }
              n217 = flat-sequence {
                tunnel: w397 -> [w439]
                tunnel: w395 -> [w437]
                tunnel: [w439] -> w401
                tunnel: [w438] -> w400
                tunnel: [w437] -> w399
                tunnel: [w436] -> w398
                tunnel: w394 -> [w436]
                tunnel: [w451] -> w396
                tunnel: w401 -> [w451]
                tunnel: w400 -> [w450]
                tunnel: w399 -> [w448]
                tunnel: w398 -> [w443]
                tunnel: [w442] -> w393
                frame #0 {
                  n218 = Get Date/Time In Seconds() -> (seconds since 1Jan1904=w438:timestamp)
                }
                frame #1 {
                  # "threshold"
                  # "delta T [ms]"
                  # "delta T [s]"
                  n219 = To Double Precision Float(number=w450) -> (double precision float=w449:dbl)
                  n220 = To Double Precision Float(number=w448) -> (double precision float=w447:dbl)
                  n221 = Subtract(x=w449, y=w447) -> (x-y=w446:dbl)
                  n222 = Multiply(x=w446, y=1000.0) -> (x*y=w441:dbl)
                  n223 = Greater?(x=w441, y=5.0) -> (0:w440:bool)
                  n224 = local write "Threshold"(w440) -> ()
                  n225 = local write "tLoop"(w441) -> ()
                  n226 = Or(x=w440, y=w443) -> (x .or. y?=w442:bool)
                }
              }
              n227 = local read "START"() -> (w418:bool)
              n228 = local read "STOP_abort"() -> (w417:bool)
              n229 = local read "Laser1_LED"() -> (w355:bool)
              n230 = local read "Laser2_LED"() -> (w354:bool)
              n231 = call "BRig_RT_panel_manualTriggering_v0,90.vi"("input_dataMTrig"=w382) -> ("output_Solenoid_R"=w385:bool, "output_Solenoid_L"=w386:bool, "output_dataMTrig"=w392:u16[], "output_Audio_L"=w387:bool, "output_Audio_R"=w388:bool, "output_CueLed"=w389:bool, "output_Laser_l1"=w390:bool, "output_Laser_l2"=w391:bool)  [unwired: 11 in]
              n232 = Or(x=w418, y=w417) -> (x .or. y?=w416:bool)
              n233 = Select(t=myRIO_BRig_RT__Case_NonExp_stateList."End" ("Enum"), s=w416, f=w415) -> (s? t:f=w414:T1)
              n234 = xnode "Read/Write Control"("FPGA VI Reference In"=w409, "error in"=w408, "A1_SR"=w385, "A3_SL"=w386, "audioTrigger_L"=w387, "audioTrigger_R"=w388, "LC_Laser_l1"=w390, "LC_Laser_l2"=w391, "CueLed_Event"=w389, "L1Led_ON"=w355, "L2Led_ON"=w354) -> ("FPGA VI Reference Out"=w420:refnum<k20>, "error out"=w397:errorcluster)
              n235 = node-c288() -> ()  [unwired: 1 in, 1 out]
            }
            n236 = node-c288(w349) -> ()  [unwired: 1 out]
            n237 = flat-sequence {
              tunnel: w343 -> [w353]
              tunnel: [w353] -> w342
              tunnel: w341 -> [w352]
              tunnel: [w352] -> w340
              frame #0 {
                w351 = FALSE
                n238 = local write "STOP_endBlock"(w351) -> ()
                n239 = local write "STOP_endTrial"(w351) -> ()
              }
            }
          }
          frame True {
            w852 = ".csv" ("string")
            w882 = ""
            w891 = u8 0
            w892 = u16 0 ("AudioLeft_phase_inc")
            w893 = FALSE
            # "Clear local files"
            # "empty array"
            # "empty array"
            # "buffer_dataBlock"
            # "buffer_dataTrial"
            # "nColumns dataBlock"
            # "nColumns dataTrial"
            # "buffer_dataBlock"
            # "buffer_dataTrial"
            # "nColumns\ndataBlock"
            # "nColumns\ndataTrial"
            # "original dataExp and dataLC"
            # "dataLick"
            # "dataTrial"
            # "dataBlock"
            # "dataCurrent"
            # "arrTrig"
            # "time stamp"
            # "dummyState counter"
            # "dataTrial"
            # "dataLick"
            # "dataLC"
            # "dataLC"
            # "dataBlock"
            # "dataMTrig"
            # "dataMTrig"
            # "dataExp"
            # "dataExp"
            # "dataCurrent"
            # "state"
            n240 = flat-sequence {
              tunnel: [w989] -> w820
              tunnel: [w988] -> w825
              tunnel: [w997] -> w839
              tunnel: [w996] -> w838
              tunnel: [myRIO_BRig_RT__Case_Exp_stateList."Start1" ("Enum")] -> w837
              tunnel: [w994] -> w836
              tunnel: [u16 0] -> w835
              tunnel: [w992] -> w834
              tunnel: [w991] -> w833
              tunnel: [w990] -> w832
              tunnel: [w999] -> w848
              tunnel: [w1000] -> w849
              tunnel: [w1001] -> w899
              tunnel: [w1002] -> w901
              tunnel: [w1003] -> w902
              tunnel: [w1004] -> w903
              tunnel: [w1005] -> w904
              tunnel: [w1006] -> w905
              tunnel: w839 -> [w1006]
              tunnel: w838 -> [w1005]
              tunnel: w837 -> [w1004]
              tunnel: w836 -> [w1003]
              tunnel: w835 -> [w1002]
              tunnel: w834 -> [w1001]
              tunnel: w833 -> [w1000]
              tunnel: w832 -> [w999]
              tunnel: [w998] -> w830
              frame #0 {
                n241 = call "BRig_dataBlock_init.vi"() -> ("output_nCol"=w988:i32, "output_dataBlock"=w990:u16[][])  [unwired: 10 in]
                n242 = call "BRig_dataCurrent_init.vi"() -> ("output_dataCurrent"=w997:u16[])  [unwired: 11 in]
                n243 = call "BRig_dataLick_init.vi"() -> ("output_dataLick"=w996:u16[][])  [unwired: 11 in]
                n244 = call "BRig_dataTrial_init.vi"() -> ("output_nCol"=w989:i32, "output_dataTrial"=w991:u16[][])  [unwired: 10 in]
                n245 = Get Date/Time In Seconds() -> (seconds since 1Jan1904=w987:timestamp)
                n246 = To Double Precision Float(number=w987) -> (double precision float=w994:dbl)
                n247 = call "BRig_arrTrig_init.vi"() -> ("output_arrTrig"=w992:bool[])  [unwired: 11 in]
              }
              frame #1 {
                w998 = u32 2 ("milliseconds to wait")
                n248 = Wait (ms)(milliseconds to wait=w998) -> ()  [unwired: 1 out]
              }
            }
            n249 = call "BRig_comm_webdav_myrioFolder.vi"() -> ("output_myrioFolder"=w853:string)  [unwired: 11 in]
            n250 = flat-sequence {
              tunnel: w827 -> [w968]
              tunnel: [w968] -> w826
              tunnel: w826 -> [w977]
              tunnel: [w975] -> w808
              tunnel: [w974] -> w824
              tunnel: [w971] -> w823
              tunnel: w825 -> [w970]
              tunnel: w820 -> [w969]
              tunnel: [w977] -> w822
              tunnel: w822 -> [w979]
              tunnel: [w979] -> w821
              tunnel: w821 -> [w985]
              tunnel: w820 -> [w984]
              tunnel: [w982] -> w815
              tunnel: [w980] -> w818
              tunnel: [w985] -> w819
              tunnel: [w986] -> _
              tunnel: w819 -> [w986]
              frame #0 {
                n251 = Wait (ms)(milliseconds to wait=w968) -> ()  [unwired: 1 out]
              }
              frame #1 {
                w972 = u16 0 ("element")
                n252 = Initialize Array(w972, 8 ("dimension size")) -> (w975:u16[])
                n253 = Initialize Array(w972, 100 ("dimension size"), w969) -> (w974:u16[][])
                n254 = Initialize Array(w972, 10 ("dimension size"), w970) -> (w971:u16[][])
              }
              frame #2 {
                n255 = Wait (ms)(milliseconds to wait=w979) -> ()  [unwired: 1 out]
              }
              frame #3 {
                n256 = Increment(x=w984) -> (x+1=w981:i32)
                n257 = To Unsigned Long Integer(number=w981) -> (unsigned 32bit integer=w980:u32)
                n258 = Initialize Array(u16 0 ("element"), w981) -> (w982:u16[])
              }
              frame #4 {
                n259 = Wait (ms)(milliseconds to wait=w986) -> ()  [unwired: 1 out]
              }
            }
            n260 = local write "stop_TimedLoop"(FALSE ("stop_TimedLoop")) -> ()
            n261 = RT FIFO Create(0:"dataTrialOrBlock" ("name (unnamed)"), 1:w815, 4:u32 40 ("size (10)"), 6:w818, 7:T8 {"read mode"=enum."blocking", "write mode"=enum."blocking"} ("r/w modes (polling,polling)")) -> (8:w817:refnum<k33>, 11:w816:errorcluster)  [unwired: 3 in, 1 out]
            n262 = RT FIFO Create(0:"dataAnalog" ("name (unnamed)"), 1:u16 0 ("element"), 4:u32 1000 ("size (10)")) -> (8:w803:refnum<k33>, 11:w802:errorcluster)  [unwired: 5 in, 1 out]
            n263 = Concatenate Strings(w853, "dataTrial" ("input_filename"), w852) -> (w854:string)
            n264 = Concatenate Strings(w853, "dataBlock" ("input_filename"), w852) -> (w855:string)
            n265 = String To Path(string=w854) -> (path=w858:path)
            n266 = String To Path(string=w855) -> (path=w850:path)
            n267 = flat-sequence {
              tunnel: [w1007] -> w831
              tunnel: w830 -> [w1007]
              tunnel: w831 -> [w1008]
              tunnel: [w1008] -> w828
              tunnel: w845 -> [w1011]
              tunnel: w796 -> [w1010]
              tunnel: [w1009] -> w829
              tunnel: w828 -> [w1009]
              tunnel: [w1015] -> _
              tunnel: w844 -> [w1015]
              tunnel: w843 -> [w1014]
              tunnel: w842 -> [w1013]
              tunnel: [w1012] -> w827
              tunnel: w829 -> [w1012]
              frame #0 {
                n268 = call "BRig_RT__Case_Exp__clearLocalFolder.vi"() -> ()  [unwired: 12 in]
              }
              frame #1 {
                n269 = Wait (ms)(milliseconds to wait=w1008) -> ()  [unwired: 1 out]
              }
              frame #2 {
                n270 = call "BRig_RT__Case_Exp__State_start__sendExpData_saveData.vi"("input_dataLC"=w1011, "input_dataExp"=w1010) -> ()  [unwired: 10 in]
              }
              frame #3 {
                n271 = call "BRig_RT__Case_Exp__State_start__sendExpData_uploadData__v2.vi"("input_error"=w1015, "input_hSession"=w1014, "input_connected"=w1013) -> ()  [unwired: 8 in, 1 out]
              }
            }
            n272 = call "BRig_RT__Case_Exp__comm_tcp__data_other.vi"("input_strState"=w882, "input_strAccum"=w882, "input_error"=w887, "input_hTCP"=w888, "input_I_connected_TCP"=w889) -> ("output_strAccum"=w883:string, "output_error"=w884:errorcluster, "output_hTCP"=w885:refnum<k5>, "output_I_connect_TCP"=w886:bool)  [unwired: 3 in]
            n273 = node-c288() -> (w911:T5)  [unwired: 4 in]
            n274 = timed-loop {
              timing: w911 -> [_]
              timing-out: [_] -> w910
              shift-right: [w1209] -> _
              shift-left: w903 -> [w1164]
              tunnel: w898 -> [w1253]
              tunnel: w897 -> [w1233]
              shift-right: [w1197] -> _
              shift-left: w909 -> [w1252]
              shift-right: [w1196] -> _
              shift-left: w908 -> [w1251]
              tunnel: [w1244] -> w890
              tunnel: [w1245] -> w907
              shift-right: [w1207] -> w878
              shift-left: w905 -> [w1181]
              shift-right: [w1250] -> w879
              shift-left: w796 -> [w1183]
              shift-right: [w1227] -> w881
              shift-left: w895 -> [w1184]
              shift-right: [w1248] -> _
              shift-left: w848 -> [w1249]
              shift-right: [w1246] -> w880
              shift-left: w845 -> [w1247]
              shift-right: [w1203] -> w877
              shift-left: w904 -> [w1210]
              shift-right: [w1243] -> _
              shift-left: w849 -> [w1182]
              tunnel: w902 -> [w1242]
              shift-right: [w1216] -> _
              shift-left: u16 0 -> [w1215]
              shift-right: [w1236] -> _
              shift-left: w901 -> [w1237]
              shift-right: [w1234] -> _
              shift-left: w899 -> [w1235]
              shift-right: [w1228] -> _
              shift-left: FALSE -> [w1230]
              shift-right: [w1172] -> w869
              shift-left: w886 -> [w1191]
              shift-right: [w1171] -> w868
              shift-left: w885 -> [w1190]
              shift-right: [w1169] -> w867
              shift-left: w884 -> [w1189]
              shift-right: [w1170] -> _
              shift-left: w883 -> [w1188]
              shift-right: [w1178] -> w874
              shift-left: w844 -> [w1178]
              shift-right: [w1180] -> w872
              shift-left: w842 -> [w1180]
              shift-right: [w1179] -> w873
              shift-left: w843 -> [w1179]
              shift-right: [w1177] -> _
              shift-left: _ -> [w1175]
              shift-right: [w1176] -> _
              shift-left: _ -> [w1174]
              tunnel: [w1173] -> w861
              tunnel: w817 -> [w1167]
              tunnel: w816 -> [w1166]
              tunnel: w815 -> [w1165]
              tunnel: w803 -> [w1163]
              tunnel: w802 -> [w1162]
              tunnel: w796 -> [w1161]
              stop <- w1173 stop-if-true
              # "iOccurrence"
              # "index"
              # "resetOccurrence?\ndataAnalog"
              # "dataLick"
              # "dataLick"
              # "dummyState counter"
              # "dummyState counter"
              # "iOccurrence"
              # "arrTrig"
              # "arrTrig"
              # "CueLed"
              # "LC_Laser_l2"
              # "LC_Event_l2"
              # "LC_Laser_l1"
              # "LC_Event_l1"
              # "iState"
              # "dataAnalog"
              # "index"
              # "manual triggering"
              # "dataTrial"
              # "dataBlock"
              # "dataExp"
              # "dataCurrent"
              # "time stamp"
              # "audio__L\naudio__R"
              # "dataLC"
              # "solenoid__R"
              # "solenoid__L"
              # "Did a lick occur?"
              # "Update lick counter"
              # "state"
              # "state"
              n275 = node-c288() -> ()  [unwired: 1 in, 1 out]
              n276 = local write "cState"(w1164) -> ()
              n277 = flat-sequence {
                tunnel: w1233 -> [w1254]
                tunnel: [w1255] -> w1231
                tunnel: [w1254] -> w1232
                frame #0 {
                  n278 = Get Date/Time In Seconds() -> (seconds since 1Jan1904=w1255:timestamp)
                }
              }
              n279 = xnode "Read/Write Control"("FPGA VI Reference In"=w1253, "error in"=w1232) -> ("FPGA VI Reference Out"=w1239:refnum<k20>, "error out"=w1238:errorcluster, "A2_LickL"=w1197:u32, "A4_LickR"=w1196:u32)
              n280 = local write "A2"(w1197) -> ()
              n281 = local write "A4"(w1196) -> ()
              n282 = Greater?(x=w1197, y=w1252) -> (0:w1205:bool)
              n283 = Greater?(x=w1196, y=w1251) -> (0:w1204:bool)
              n284 = Or(x=w1205, y=w1204) -> (x .or. y?=w1206:bool)
              n285 = case shown="\"endTrial1\"" w1164 {
                selector: w1164 -> [_ _ _ _ _ _ _ _ _ _ _ _ _ w1455 _ w1484 _ w1516 _ w1542 _ w1586 _ w1626 _ w1646 _ w1684 _ w1726 _ _ _ _ w1845 _ w1869 w1900 w1921 w1946 _ w2003 w2013 _]
                tunnel: [myRIO_BRig_RT__Case_Exp_stateList."Start2" ("Enum") myRIO_BRig_RT__Case_Exp_stateList."Start3" ("Enum") myRIO_BRig_RT__Case_Exp_stateList."saveSettings1" ("Enum") myRIO_BRig_RT__Case_Exp_stateList."initBlock" ("Enum") myRIO_BRig_RT__Case_Exp_stateList."initTrial_LC_ENL1" ("Enum") myRIO_BRig_RT__Case_Exp_stateList."initTrial" ("Enum") myRIO_BRig_RT__Case_Exp_stateList."initTrial2" ("Enum") myRIO_BRig_RT__Case_Exp_stateList."setSettings_Laser" ("Enum") myRIO_BRig_RT__Case_Exp_stateList."ENL1_pre" ("Enum") myRIO_BRig_RT__Case_Exp_stateList."initTrial_LC_Cue1" ("Enum") myRIO_BRig_RT__Case_Exp_stateList."initTrial_LC_Sel" ("Enum") myRIO_BRig_RT__Case_Exp_stateList."initTrial4" ("Enum") w1445 w1453 myRIO_BRig_RT__Case_Exp_stateList."ENL1Penalty" ("Enum") w1482 w1496 w1515 myRIO_BRig_RT__Case_Exp_stateList."Cue1Penalty" ("Enum") w1543 w1559 w1581 myRIO_BRig_RT__Case_Exp_stateList."SelectReward" ("Enum") w1625 myRIO_BRig_RT__Case_Exp_stateList."SelectRewardPost" ("Enum") w1645 myRIO_BRig_RT__Case_Exp_stateList."SelectWrong" ("Enum") w1683 myRIO_BRig_RT__Case_Exp_stateList."SelectTimeout" ("Enum") w1725 myRIO_BRig_RT__Case_Exp_stateList."saveData_dataTrial" ("Enum") w1760 w1795 w1834 w1845 myRIO_BRig_RT__Case_Exp_stateList."initBlock" ("Enum") w1867 w1901 w1920 w1945 myRIO_BRig_RT__Case_Exp_stateList."FreeReward" ("Enum") w2001 w2011 myRIO_BRig_RT__Case_Exp_stateList."FreeRewardPost" ("Enum")] -> w1209
                tunnel: w1206 -> [_ _ _ _ _ _ _ _ _ _ _ _ w1446 w1454 _ _ w1497 w1517 _ _ _ _ _ _ _ _ _ _ _ _ _ _ _ _ _ _ _ _ _ _ _ _ _ _]
                tunnel: w1205 -> [_ _ _ _ _ _ _ _ _ _ _ _ _ _ _ _ _ _ _ _ w1551 w1582 _ _ _ _ _ _ _ _ _ _ _ _ _ _ _ _ _ _ _ _ _ _]
                tunnel: w1204 -> [_ _ _ _ _ _ _ _ _ _ _ _ _ _ _ _ _ _ _ _ w1550 w1583 _ _ _ _ _ _ _ _ _ _ _ _ _ _ _ _ _ _ _ _ _ _]
                tunnel: w1181 -> [w1265 w1271 w1286 w1290 w1311 w1348 w1351 w1366 w1393 w1408 w1418 w1435 w1443 w1462 w1473 w1481 w1498 w1518 w1535 w1541 w1562 w1579 w1611 w1622 w1634 w1644 w1668 w1682 w1706 w1724 w1739 w1766 w1804 w1824 w1844 w1851 w1870 w1903 w1919 w1936 w1975 w1999 w2010 w2021]
                tunnel: w1183 -> [w1256 w1270 w1276 w1288 w1299 w1347 w1361 w1367 w1404 w1407 w1417 w1427 w1450 w1465 w1472 w1489 w1495 w1521 w1528 w1549 w1558 w1578 w1613 w1624 w1632 w1651 w1664 w1689 w1701 w1731 w1749 w1758 w1802 w1809 w1843 w1848 w1872 w1905 w1931 w1951 w1956 w2004 w2014 w2020]
                tunnel: [w1265 w1271 w1286 w1290 w1311 w1346 w1350 w1369 w1393 w1411 w1425 w1434 w1447 w1461 w1474 w1480 w1492 w1501 w1534 w1540 w1557 w1580 w1604 w1627 w1633 w1642 w1661 w1680 w1699 w1723 w1741 w1766 w1804 w1824 w1844 w1851 w1870 w1903 w1919 w1936 w1981 w2000 w2009 w2019] -> w1208
                tunnel: [w1256 w1270 w1275 w1288 w1299 w1347 w1361 w1367 w1404 w1407 w1417 w1427 w1450 w1465 w1472 w1489 w1495 w1521 w1528 w1549 w1558 w1578 w1613 w1624 w1632 w1651 w1664 w1689 w1701 w1731 w1749 w1755 w1802 w1808 w1843 w1848 w1872 w1905 w1931 w1951 w1957 w2004 w2014 w2020] -> w1250
                tunnel: [_ _ _ _ _ _ _ _ _ _ _ _ _ _ _ _ _ _ _ _ _ _ _ w1616 _ _ _ _ _ _ _ _ _ _ _ _ _ _ _ _ _ w1993 _ _] -> w1193
                tunnel: [_ _ _ _ _ _ _ _ _ _ _ _ _ _ _ _ _ _ _ _ _ _ _ w1615 _ _ _ _ _ _ _ _ _ _ _ _ _ _ _ _ _ w1994 _ _] -> w1192
                tunnel: w1249 -> [w1264 w1268 w1284 w1292 w1324 w1343 w1355 w1383 w1405 w1413 w1424 w1432 w1449 w1464 w1469 w1487 w1500 w1520 w1533 w1546 w1568 w1590 w1610 w1629 w1638 w1649 w1666 w1687 w1705 w1730 w1735 w1767 w1793 w1826 w1841 w1850 w1852 w1906 w1929 w1949 w1984 w2006 w2016 w2028]
                tunnel: [w1264 w1268 w1284 w1292 w1324 w1342 w1354 w1383 w1405 w1413 w1424 w1432 w1449 w1464 w1469 w1487 w1500 w1520 w1533 w1546 w1568 w1590 w1609 w1629 w1638 w1649 w1665 w1687 w1703 w1730 w1735 w1767 w1793 w1826 w1841 w1850 w1852 w1906 w1929 w1949 w1984 w2006 w2016 w2028] -> w1248
                tunnel: w1247 -> [w1257 w1269 w1285 w1291 w1319 w1349 w1365 w1384 w1406 w1412 w1419 w1433 w1448 w1463 w1470 w1488 w1499 w1519 w1532 w1548 w1567 w1591 w1612 w1628 w1641 w1650 w1670 w1688 w1712 w1729 w1748 w1757 w1805 w1828 w1842 w1847 w1871 w1904 w1930 w1950 w1985 w2007 w2017 w2029]
                tunnel: [w1257 w1269 w1285 w1291 w1319 w1349 w1365 w1384 w1406 w1412 w1419 w1433 w1448 w1463 w1470 w1488 w1499 w1519 w1532 w1548 w1567 w1591 w1612 w1628 w1641 w1650 w1670 w1688 w1712 w1729 w1748 w1756 w1805 w1828 w1842 w1847 w1871 w1904 w1930 w1950 w1985 w2007 w2017 w2029] -> w1246
                tunnel: [_ _ _ _ _ _ _ _ _ _ _ _ _ _ _ _ _ _ _ _ _ _ _ _ _ _ _ _ _ _ _ _ _ _ TRUE _ _ _ _ _ _ _ _ _] -> w1211
                tunnel: [_ _ _ _ _ _ _ _ _ _ _ _ _ _ _ _ _ w1503 _ _ _ _ _ _ _ _ _ _ _ _ _ _ _ _ _ _ _ _ _ _ _ _ _ _] -> w1241
                tunnel: [_ _ _ _ _ _ _ _ _ _ _ _ _ _ _ _ _ w1502 _ _ _ _ _ _ _ _ _ _ _ _ _ _ _ _ _ _ _ _ _ _ _ _ _ _] -> w1240
                tunnel: w1182 -> [w1262 w1267 w1282 w1289 w1323 w1341 w1360 w1385 w1397 w1414 w1423 w1431 w1442 w1452 w1466 w1486 w1494 w1506 w1530 w1545 w1566 w1570 w1601 w1623 w1639 w1648 w1663 w1686 w1704 w1728 w1747 w1765 w1803 w1825 w1839 w1849 w1856 w1883 w1928 w1948 w1979 w2005 w2015 w2027]
                tunnel: [w1262 w1267 w1282 w1289 w1323 w1340 w1353 w1368 w1391 w1410 w1422 w1430 w1441 w1451 w1466 w1486 w1493 w1505 w1530 w1545 w1566 w1569 w1600 w1623 w1639 w1648 w1660 w1686 w1698 w1728 w1746 w1765 w1803 w1825 w1839 w1849 w1856 w1883 w1928 w1948 w1979 w2005 w2015 w2027] -> w1243
                tunnel: w1242 -> [_ _ _ _ _ _ _ _ _ _ _ _ _ _ _ _ _ _ _ _ _ _ _ _ _ _ _ _ _ _ w1740 _ _ _ _ _ _ _ _ _ _ _ _ _]
                tunnel: w1239 -> [w1261 _ _ _ w1320 w1335 w1364 w1389 w1402 _ _ w1438 _ _ _ _ _ w1507 _ _ w1564 w1589 w1599 _ _ _ _ _ w1710 _ w1743 _ _ _ w1837 _ _ _ _ _ w1963 _ _ _]
                tunnel: w1238 -> [w1260 _ _ _ w1321 w1334 w1352 w1388 w1401 _ _ w1437 _ _ _ _ _ w1508 _ _ w1565 w1588 w1598 _ _ _ _ _ w1709 _ w1742 _ _ _ w1836 _ _ _ _ _ w1962 _ _ _]
                tunnel: [_ _ _ _ _ _ _ _ _ _ _ _ _ w1460 _ _ _ w1513 _ _ w1556 w1576 _ _ _ _ _ _ _ _ _ _ _ _ _ _ _ _ _ _ _ _ _ _] -> w1217
                tunnel: [_ _ _ _ _ _ _ _ _ _ _ _ _ w1459 _ _ _ w1512 _ _ w1555 w1575 _ _ _ _ _ _ _ _ _ _ _ _ _ _ _ _ _ _ _ _ _ _] -> w1198
                tunnel: [_ _ _ _ _ _ _ _ TRUE ("Recording") _ _ _ _ _ _ _ _ _ _ _ _ _ _ _ _ _ _ _ _ _ _ _ _ _ _ _ _ _ _ _ _ _ _ _] -> w1214
                tunnel: w1237 -> [_ _ _ _ _ _ _ _ _ _ _ _ _ _ _ _ _ _ _ _ _ _ _ _ _ _ _ _ _ _ _ _ _ _ _ _ w1868 w1899 w1926 w1933 _ _ _ _]
                tunnel: [_ _ _ _ _ _ _ _ _ _ _ _ _ _ _ _ _ _ _ _ _ _ _ _ _ _ _ _ _ _ _ _ _ _ _ _ w1866 w1898 w1924 w1934 _ _ _ _] -> w1236
                tunnel: w1235 -> [_ _ _ _ w1293 _ _ _ w1398 w1415 w1421 w1429 w1444 w1456 w1467 w1485 w1491 w1514 w1529 w1544 w1552 w1577 _ _ _ _ _ _ _ _ _ _ _ _ _ _ _ _ _ _ _ _ _ _]
                tunnel: [_ _ _ _ w1293 _ _ w1370 w1398 w1409 w1420 w1428 w1444 w1456 w1467 w1485 w1490 w1514 w1529 w1544 w1552 w1577 _ _ _ _ _ _ _ _ _ _ _ _ _ _ _ _ _ _ _ _ _ _] -> w1234
                tunnel: [_ _ _ _ _ _ _ _ _ _ _ _ _ w1458 _ _ _ w1511 _ _ w1554 w1574 _ _ _ _ _ _ _ _ _ _ _ _ _ _ _ _ _ _ _ _ _ _] -> w1221
                tunnel: [_ _ _ _ _ _ _ _ _ _ _ _ _ w1457 _ _ _ w1510 _ _ w1553 w1573 _ _ _ _ _ _ _ _ _ _ _ _ _ _ _ _ _ _ _ _ _ _] -> w1222
                tunnel: [_ _ _ _ _ _ _ _ _ _ _ _ _ _ _ _ _ w1504 _ _ _ _ _ _ _ _ _ _ _ _ _ _ _ _ _ _ _ _ _ _ _ _ _ _] -> w1224
                tunnel: [_ _ "<S,S>" ("string") _ _ _ _ _ w1392 _ _ _ _ _ _ _ _ _ _ _ _ _ w1602 _ _ _ w1659 _ w1697 _ w1738 _ _ w1820 _ _ _ _ _ _ _ _ _ _] -> w1187
                tunnel: w1184 -> [_ _ _ _ _ _ _ _ _ _ _ _ _ _ _ _ _ _ _ _ _ _ _ _ _ _ _ _ _ _ _ _ _ _ _ _ _ _ _ _ w1970 _ _ _]
                tunnel: w1180 -> [_ _ _ _ _ _ _ _ _ _ _ _ _ _ _ _ _ _ _ _ _ _ _ _ _ _ _ _ _ _ _ _ _ w1819 _ _ _ _ _ _ _ _ _ _]
                tunnel: w1179 -> [_ _ _ _ _ _ _ _ _ _ _ _ _ _ _ _ _ _ _ _ _ _ _ _ _ _ _ _ _ _ _ _ _ _ _ _ _ _ _ _ _ _ _ _]
                tunnel: w1178 -> [_ _ _ _ _ _ _ _ _ _ _ _ _ _ _ _ _ _ _ _ _ _ _ _ _ _ _ _ _ _ _ _ _ _ _ _ _ _ _ _ _ _ _ _]
                tunnel: [_ _ _ _ _ _ _ _ _ _ _ _ _ _ _ _ _ _ _ _ _ _ _ _ _ _ _ _ _ _ _ w1759 _ _ _ _ _ _ _ _ _ _ _ _] -> w1177
                tunnel: [_ _ _ _ _ _ _ _ _ _ _ _ _ _ _ _ _ _ _ _ _ _ _ _ _ _ _ _ _ _ _ w1764 _ _ _ _ _ _ _ _ _ _ _ _] -> w1176
                tunnel: w1175 -> [_ _ _ _ _ _ _ _ _ _ _ _ _ _ _ _ _ _ _ _ _ _ _ _ _ _ _ _ _ _ _ w1763 _ _ _ _ _ _ _ _ _ _ _ _]
                tunnel: w1174 -> [_ _ _ _ _ _ _ _ _ _ _ _ _ _ _ _ _ _ _ _ _ _ _ _ _ _ _ _ _ _ _ w1754 _ _ _ _ _ _ _ _ _ _ _ _]
                tunnel: w1167 -> [_ _ _ _ _ _ _ _ _ _ _ _ _ _ _ _ _ _ _ _ _ _ _ _ _ _ _ _ _ _ _ _ _ _ _ _ w1863 w1886 _ _ _ _ _ _]
                tunnel: w1166 -> [_ _ _ _ _ _ _ _ _ _ _ _ _ _ _ _ _ _ _ _ _ _ _ _ _ _ _ _ _ _ _ _ _ _ _ _ w1862 w1885 _ _ _ _ _ _]
                tunnel: w1165 -> [_ _ _ _ _ _ _ _ _ _ _ _ _ _ _ _ _ _ _ _ _ _ _ _ _ _ _ _ _ _ _ _ _ _ _ _ w1860 w1884 _ _ _ _ _ _]
                tunnel: w1161 -> [_ _ _ _ _ _ _ _ _ _ _ _ _ _ _ _ _ _ _ _ _ _ _ _ _ _ _ _ _ _ _ _ _ w1814 _ _ _ _ _ _ _ _ _ _]
                frame "Start1", Default {
                  w1259 = FALSE ("SelectionState")
                  n286 = xnode "Read/Write Control"("FPGA VI Reference In"=w1261, "error in"=w1260, "SelectionState"=w1259, "LR_reward_Laser_l1"=w1259, "LR_wrong_Laser_l1"=w1259, "LR_reward_Event_l1"=w1259, "LR_wrong_Event_l1"=w1259, "Left(F)_or_Right(T)"=w1259, "SelectionState"=w1259, "LR_reward_Laser_l2"=w1259, "LR_wrong_laser_l2"=w1259, "LR_reward_Event_l2"=w1259, "LR_wrong_Event_l2"=w1259, "LC_Event_l1"=w1259, "LC_Laser_l1"=w1259, "LC_Laser_l2"=w1259, "LC_Event_l2"=w1259, "CueLed_Event"=w1259) -> ("error out"=w1258:errorcluster)  [unwired: 1 out]
                  n287 = local write "error out"(w1258) -> ()
                }
                frame "Start2" {
                }
                frame "Start3" {
                  w1272 = u16 0 ("new element/subarray")
                  w1277 = 0.0 ("BTPR_avg_L")
                  w1280 = FALSE ("SolenoidReward")
                  w1278 = u16 0 ("BTPR_block")
                  w1281 = u16 0 ("nRewards_cur")
                  # "Goal:\nPrepare dataCurrent"
                  n288 = call "BRig_dataExp_FreeReward_c_L.vi"() -> ("output_FreeReward_c_L"=w1274:i32)  [unwired: 11 in]
                  n289 = call "BRig_dataExp_FreeReward_c_R.vi"() -> ("output_FreeReward_c_R"=w1273:i32)  [unwired: 11 in]
                  n290 = local write "nRewards_cur"(w1281) -> ()
                  n291 = local write "nRewards_total"(w1281) -> ()
                  n292 = local write "nRewards_Left"(w1281) -> ()
                  n293 = local write "nRewards_Right"(w1281) -> ()
                  n294 = local write "BUR_target"(w1281) -> ()
                  n295 = local write "TpB_target"(w1281) -> ()
                  n296 = local write "iBlock"(w1281) -> ()
                  n297 = local write "iTrial"(w1281) -> ()
                  n298 = local write "nTrial"(w1281) -> ()
                  n299 = local write "SolenoidReward"(w1280) -> ()
                  n300 = local write "allReward_L"(w1280) -> ()
                  n301 = local write "allReward_R"(w1280) -> ()
                  n302 = Replace Array Subset(array=w1276, new element #1=w1272, index #1=w1274, new element #2=w1272, index #2=w1273) -> (w1275:u16[])
                  n303 = local write "FreeReward_c_L"(w1272) -> ()
                  n304 = local write "FreeReward_c_R"(w1272) -> ()
                  n305 = local write "BTPR_block"(w1278) -> ()
                  n306 = local write "T2R_block"(w1278) -> ()
                  n307 = local write "BTPR_avg_L"(w1277) -> ()
                  n308 = local write "BTPR_avg_R"(w1277) -> ()
                  n309 = local write "T2R_avg_L"(w1277) -> ()
                  n310 = local write "T2R_avg_R"(w1277) -> ()
                }
                frame "saveSettings1" {
                }
                frame "setSettings_Laser" {
                  n311 = call "BRig_dataExp_LED_baseline_Cue.vi"() -> ("output_LED_baseline_Cue"=w1308:i32)  [unwired: 11 in]
                  n312 = call "BRig_dataExp_LED_baseline_l1.vi"() -> ("output_LED_baseline_l1"=w1309:i32)  [unwired: 11 in]
                  n313 = call "BRig_dataExp_LED_baseline_l2.vi"() -> ("output_LED_baseline_l2"=w1307:i32)  [unwired: 11 in]
                  n314 = call "BRig_dataExp_I_anySelect.vi"() -> ("output_I_anySelect"=w1301:i32)  [unwired: 11 in]
                  n315 = call "BRig_dataExp_I_trialUntilReward.vi"() -> ("output_I_trialUntilReward"=w1300:i32)  [unwired: 11 in]
                  n316 = local read "FPGA_count2ms"() -> (w1318:dbl)
                  n317 = call "BRig_RT__Case_Exp__State_setLaserSettings.vi"("input_FPGA_count2ms"=w1318, "input_dataExp"=w1299, "input_dataLC"=w1319) -> ("output_LR_nTotal_l1"=w1317:u32, "output_LR_nTotal_l2"=w1316:u32, "output_LR_reward_nDelay_l1"=w1315:u32, "output_LR_wrong_nDelay_l1"=w1314:u32, "output_LR_reward_nDelay_l2"=w1313:u32, "output_LR_wrong_nDelay_l2"=w1312:u32)  [unwired: 11 in]
                  n318 = Index Array(array=w1299, index #1=w1308, index #2=w1309, index #3=w1307, index #4=w1301, index #5=w1300) -> (element #1=w1306:u16, element #2=w1305:u16, element #3=w1304:u16, element #4=w1303:u16, element #5=w1302:u16)
                  n319 = Not Equal To 0?(x=w1305) -> (x != 0?=w1297:bool)
                  n320 = Not Equal To 0?(x=w1303) -> (x != 0?=w1295:bool)
                  n321 = Not Equal To 0?(x=w1306) -> (x != 0?=w1298:bool)
                  n322 = Not Equal To 0?(x=w1304) -> (x != 0?=w1296:bool)
                  n323 = Not Equal To 0?(x=w1302) -> (x != 0?=w1294:bool)
                  n324 = xnode "Read/Write Control"("FPGA VI Reference In"=w1320, "error in"=w1321, "LR_reward_nTotal_l1"=w1317, "LR_wrong_nTotal_l1"=w1317, "LR_reward_nTotal_l2"=w1316, "LR_wrong_nTotal_l2"=w1316, "LR_reward_nDelay_l1"=w1315, "LR_wrong_nDelay_l1"=w1314, "LR_reward_nDelay_l2"=w1313, "LR_wrong_nDelay_l2"=w1312, "CueLed_Baseline"=w1298, "L1Led_Baseline"=w1297, "L2Led_Baseline"=w1296, "I_allReward"=w1295, "ignoreWrong"=w1294) -> ("error out"=→"error out":errorcluster)  [unwired: 1 out]
                }
                frame "initBlock" {
                  w1325 = u16 0 ("BTPR_block")
                  n325 = local write "nRewards_cur"(u16 0 ("nRewards_cur")) -> ()
                  n326 = local write "BTPR_block"(w1325) -> ()
                  n327 = local write "T2R_block"(w1325) -> ()
                  n328 = call "BRig_RT__Case_Exp__State_initBlock.vi"("input_dataCurrent"=w1348, "input_dataExp"=w1347, "input_dataBlock"=w1343, "input_dataTrial"=w1341) -> ("output_iSpout"=w1332:u16, "output_speaker_amp_R"=w1336:u16, "output_iBlock"=w1331:u16, "output_speaker_freq_R"=w1337:u8, "output_BUR_target"=w1330:u16, "output_speaker_amp_L"=w1338:u16, "output_TpB_target"=w1345:u16, "output_speaker_freq_L"=w1339:u8, "output_dataCurrent"=w1346:u16[], "output_dataBlock"=w1342:u16[][], "output_dataTrial"=w1340:u16[][])  [unwired: 5 in]
                  n329 = Type Cast(type=enum16{"Left", "Right"}."Left", x=w1332) -> (*(type *) &x=w1327:enum16{"Left", "Right"})
                  n330 = Not Equal To 0?(x=w1332) -> (x != 0?=w1326:bool)
                  n331 = local write "cSpout"(w1327) -> ()
                  n332 = local write "iBlock"(w1331) -> ()
                  n333 = local write "BUR_target"(w1330) -> ()
                  n334 = local write "TpB_target"(w1345) -> ()
                  n335 = xnode "Read/Write Control"("FPGA VI Reference In"=w1335, "error in"=w1334, "Left(F)_or_Right(T)"=w1326, "audioFreq_L_kHz"=w1339, "audioAmp_L"=w1338, "audioFreq_R_kHz"=w1337, "audioAmp_R"=w1336) -> ("error out"=w1333:errorcluster)  [unwired: 1 out]
                  n336 = local write "error out"(w1333) -> ()
                }
                frame "initTrial" {
                  n337 = xnode "Read/Write Control"("FPGA VI Reference In"=w1364, "error in"=w1352, "SelectionState"=FALSE) -> ("error out"=w1363:errorcluster)  [unwired: 1 out]
                  n338 = call "BRig_RT__Case_Exp__State_initTrial__v2.vi"("input_dataCurrent"=w1351, "input_dataBlock"=w1355, "input_dataTrial"=w1360, "input_dataExp"=w1361) -> ("output_iTrial"=w1358:u16, "output_nTrial"=w1356:u16, "output_SolenoidReward"=w1359:bool, "output_dataCurrent"=w1350:u16[], "output_dataBlock"=w1354:u16[][], "output_dataTrial"=w1353:u16[][])  [unwired: 6 in]
                  n339 = local write "iTrial"(w1358) -> ()
                  n340 = local write "nTrial"(w1356) -> ()
                  n341 = local write "SolenoidReward"(w1359) -> ()
                  n342 = local write "error out"(w1363) -> ()
                }
                frame "initTrial2" {
                  n343 = call "BRig_RT__Case_Exp__State_initTrial2.vi"("input_dataCurrent"=w1366, "input_dataTrial"=w1385, "input_dataExp"=w1367, "input_dataBlock"=w1383, "input_dataLC"=w1384) -> ("output_L_Wrong_Laser_l2"=w1375:bool, "output_L_Wrong_Event_l2"=w1376:bool, "output_L_Power_l1"=w1374:dbl, "output_L_Reward_Laser_l2"=w1377:bool, "output_L_Power_l2"=w1373:dbl, "output_L_Reward_Event_l2"=w1378:bool, "output_dataCurrent"=w1369:u16[], "output_dataTrial"=w1368:u16[][], "output_L_Reward_Event_l1"=w1382:bool, "output_L_Reward_Laser_l1"=w1381:bool, "output_L_Wrong_Event_l1"=w1380:bool, "output_L_Wrong_Laser_l1"=w1379:bool)  [unwired: 3 in]
                  n344 = local write "L_Power_l1"(w1374) -> ()
                  n345 = call "myRIO__convert__Voltage_to_FPGAvalue.vi"("input_voltage"=w1374) -> ("output_PortC"=w1371:i16)  [unwired: 9 in, 1 out]
                  n346 = local write "L_Power_l2"(w1373) -> ()
                  n347 = call "myRIO__convert__Voltage_to_FPGAvalue.vi"("input_voltage"=w1373) -> ("output_PortC"=w1372:i16)  [unwired: 9 in, 1 out]
                  n348 = xnode "Read/Write Control"("FPGA VI Reference In"=w1389, "error in"=w1388, "AnaOut_0"=w1371, "AnaOut_1"=w1372, "LR_reward_Event_l1"=w1382, "LR_reward_Laser_l1"=w1381, "LR_wrong_Event_l1"=w1380, "LR_wrong_Laser_l1"=w1379, "LR_reward_Event_l2"=w1378, "LR_reward_Laser_l2"=w1377, "LR_wrong_Event_l2"=w1376, "LR_wrong_laser_l2"=w1375) -> ("error out"=w1386:errorcluster)  [unwired: 1 out]
                  n349 = local write "error out"(w1386) -> ()
                  n350 = call "BRig_arrTrig_init.vi"() -> ("output_arrTrig"=w1370:bool[])  [unwired: 11 in]
                }
                frame "initTrial4" {
                  # "resetOccurrence?\ndataAnalog"
                  n351 = local read "FPGA_count2ms"() -> (w1394:dbl)
                  n352 = local read "lick_Rising(F)_or_Falling(T)"() -> (w1390:bool)
                  n353 = local read "Recording"() -> (w1396:bool)
                  n354 = call "BRig_RT_comm_tcp_write_RTwrite__RunState_Trial_start.vi"("input_dataCurrent"=w1393) -> ("output_strCmd"=w1392:string)  [unwired: 10 in]
                  n355 = call "BRig_RT__Case_Exp__State_initTrial4.vi"("input_Recording"=w1396, "input_FPGA_count2ms"=w1394, "input_dataTrial"=w1397) -> ("output_Solenoid_nTotal"=w1395:u32, "output_dataTrial"=w1391:u16[][])  [unwired: 7 in]
                  n356 = xnode "Read/Write Control"("FPGA VI Reference In"=w1402, "error in"=w1401, "Solenoid_nTotal_L"=w1395, "Solenoid_nTotal_R"=w1395, "A6_Act"=w1396, "Rising(F)_or_Falling(T)"=w1390) -> ("error out"=w1400:errorcluster)  [unwired: 1 out]
                  n357 = local write "error out"(w1400) -> ()
                }
                frame "initTrial_LC_ENL1" {
                  n358 = call "BRig_RT__Case_Exp__State_initTrial__LC_ENL.vi"("input_arrTrig"=w1415, "input_dataTrial"=w1414, "input_dataExp"=w1407, "input_dataLC"=w1412, "input_dataCurrent"=w1408) -> ("output_dataTrial"=w1410:u16[][], "output_dataCurrent"=w1411:u16[], "output_arrTrig"=w1409:bool[])  [unwired: 4 in]
                }
                frame "initTrial_LC_Cue1" {
                  n359 = call "BRig_RT__Case_Exp__State_initTrial__LC_Cue.vi"("input_arrTrig"=w1421, "input_dataTrial"=w1423, "input_dataExp"=w1417, "input_dataLC"=w1419, "input_dataCurrent"=w1418) -> ("output_dataTrial"=w1422:u16[][], "output_dataCurrent"=w1425:u16[], "output_arrTrig"=w1420:bool[])  [unwired: 4 in]
                }
                frame "initTrial_LC_Sel" {
                  n360 = call "BRig_RT__Case_Exp__State_initTrial__LC_Select.vi"("input_arrTrig"=w1429, "input_dataTrial"=w1431, "input_dataExp"=w1427, "input_dataLC"=w1433, "input_dataCurrent"=w1435) -> ("output_dataTrial"=w1430:u16[][], "output_dataCurrent"=w1434:u16[], "output_arrTrig"=w1428:bool[])  [unwired: 4 in]
                  n361 = xnode "Read/Write Control"("FPGA VI Reference In"=w1438, "error in"=w1437, "A6_Act"=FALSE) -> ("error out"=w1439:errorcluster)  [unwired: 1 out]
                  n362 = local write "error out"(w1439) -> ()
                }
                frame "ENL1_pre" {
                  n363 = call "BRig_RT__Case_Exp__State_ENLPre.vi"("input_I_lick"=w1446, "input_dataTrial"=w1442, "input_dataCurrent"=w1443) -> ("output_dataTrial"=w1441:u16[][], "output_dataCurrent"=w1447:u16[], "output_state"=w1445:T2)  [unwired: 6 in]
                }
                frame "ENL1" {
                  n364 = call "BRig_RT__Case_Exp__State_ENL.vi"("input_dataCurrent"=w1462, "input_dataTrial"=w1452, "input_arrTrig"=w1456, "input_state"=w1455, "I_lick"=w1454) -> ("output_l2_laserOn"=w1457:bool, "output_l2_laserEvent"=w1458:bool, "output_l1_laserOn"=w1459:bool, "output_state"=w1453:T2, "output_l1_laserEvent"=w1460:bool, "output_dataCurrent"=w1461:u16[], "output_dataTrial"=w1451:u16[][])  [unwired: 8 in]
                }
                frame "ENL1Penalty_pre" {
                  n365 = call "BRig_dataCurrent_c_generic.vi"() -> ("output_count_generic"=w1478:i32)  [unwired: 11 in]
                  n366 = call "BRig_dataCurrent_T_generic.vi"() -> ("output_T_generic"=w1476:i32)  [unwired: 11 in]
                  n367 = call "BRig_dataExp_T_ENLPenalty.vi"() -> ("output_ENL_penalty"=w1471:i32)  [unwired: 11 in]
                  n368 = Index Array(array=w1472, index=w1471) -> (element=w1475:u16)
                  n369 = Replace Array Subset(array=w1473, new element #1=u16 0 ("new element/subarray"), index #1=w1478, new element #2=w1475, index #2=w1476) -> (w1474:u16[])
                }
                frame "ENL1Penalty" {
                  n370 = call "BRig_RT__Case_Exp__generic__incrementCountTilThreshold.vi"("input_dataCurrent"=w1481) -> ("output_dataCurrent"=w1480:u16[], "output_underThreshold"=w1479:bool)  [unwired: 9 in]
                  n371 = Select(t=w1484, s=w1479, f=myRIO_BRig_RT__Case_Exp_stateList."ENL1_pre" ("Enum")) -> (s? t:f=w1482:T2)
                }
                frame "Cue1_pre" {
                  n372 = call "BRig_RT__Case_Exp__State_CuePre.vi"("input_dataCurrent"=w1498, "input_dataTrial"=w1494, "input_I_lick"=w1497, "input_dataExp"=w1495, "input_arrTrig"=w1491) -> ("output_state"=w1496:T2, "output_arrTrig"=w1490:bool[], "output_dataCurrent"=w1492:u16[], "output_dataTrial"=w1493:u16[][])  [unwired: 11 in]
                }
                frame "Cue1" {
                  n373 = call "BRig_RT__Case_Exp__State_Cue.vi"("input_dataCurrent"=w1518, "input_dataTrial"=w1506, "input_arrTrig"=w1514, "input_state"=w1516, "I_lick"=w1517) -> ("output_l2_laserOn"=w1510:bool, "output_l2_laserEvent"=w1511:bool, "output_SelectionState"=w1509:bool, "output_l1_laserOn"=w1512:bool, "output_state"=w1515:T2, "output_l1_laserEvent"=w1513:bool, "output_dataCurrent"=w1501:u16[], "output_dataTrial"=w1505:u16[][], "output_CueLed"=w1504:bool, "output_Audio_L"=w1503:bool, "output_Audio_R"=w1502:bool)  [unwired: 4 in]
                  n374 = case shown="True" w1509 {
                    selector: w1509 -> [_ w1524]
                    tunnel: w1508 -> [_ w1523]
                    tunnel: w1507 -> [_ w1522]
                    frame False {
                    }
                    frame True {
                      n375 = xnode "Read/Write Control"("FPGA VI Reference In"=w1522, "error in"=w1523, "SelectionState"=w1524) -> ("error out"=w1525:errorcluster)  [unwired: 1 out]
                      n376 = local write "error out"(w1525) -> ()
                    }
                  }
                }
                frame "Cue1Penalty_pre" {
                  n377 = call "BRig_dataCurrent_c_generic.vi"() -> ("output_count_generic"=w1538:i32)  [unwired: 11 in]
                  n378 = call "BRig_dataCurrent_T_generic.vi"() -> ("output_T_generic"=w1536:i32)  [unwired: 11 in]
                  n379 = call "BRig_dataExp_T_CuePenalty.vi"() -> ("output_T_CuePenalty"=w1527:i32)  [unwired: 11 in]
                  n380 = Index Array(array=w1528, index=w1527) -> (element=w1526:u16)
                  n381 = Replace Array Subset(array=w1535, new element #1=u16 0 ("new element/subarray"), index #1=w1538, new element #2=w1526, index #2=w1536) -> (w1534:u16[])
                }
                frame "Cue1Penalty" {
                  n382 = call "BRig_RT__Case_Exp__generic__incrementCountTilThreshold.vi"("input_dataCurrent"=w1541) -> ("output_dataCurrent"=w1540:u16[], "output_underThreshold"=w1539:bool)  [unwired: 9 in]
                  n383 = Select(t=w1542, s=w1539, f=myRIO_BRig_RT__Case_Exp_stateList."ENL1_pre" ("Enum")) -> (s? t:f=w1543:T2)
                }
                frame "Selection_pre" {
                  n384 = xnode "Read/Write Control"("FPGA VI Reference In"=w1564, "error in"=w1565) -> ("error out"=w1563:errorcluster, "SelectReward"=w1560:bool, "SelectWrong"=w1561:bool)  [unwired: 1 out]
                  n385 = call "BRig_RT__Case_Exp__State_SelectPre.vi"("input_dataCurrent"=w1562, "input_SelectWrong"=w1561, "input_SelectReward"=w1560, "input_dataExp"=w1558, "input_LickL"=w1551, "input_LickR"=w1550, "input_arrTrig"=w1552) -> ("output_state"=w1559:T2, "output_dataCurrent"=w1557:u16[], "output_l1_laserEvent"=w1556:bool, "output_l1_laserOn"=w1555:bool, "output_l2_laserOn"=w1553:bool, "output_l2_laserEvent"=w1554:bool)  [unwired: 3 in]
                  n386 = local write "error out"(w1563) -> ()
                }
                frame "Selection" {
                  n387 = xnode "Read/Write Control"("FPGA VI Reference In"=w1589, "error in"=w1588) -> ("error out"=w1587:errorcluster, "SelectReward"=w1584:bool, "SelectWrong"=w1585:bool)  [unwired: 1 out]
                  n388 = call "BRig_RT__Case_Exp__State_Selection.vi"("input_state"=w1586, "input_dataCurrent"=w1579, "input_dataTrial"=w1570, "input_dataExp"=w1578, "input_arrTrig"=w1577, "input_FPGA_SelectWrong"=w1585, "input_FPGA_SelectReward"=w1584, "input_LickR"=w1583, "input_LickL"=w1582) -> ("output_LC_Laser_l2"=w1573:bool, "output_LC_Event_l2"=w1574:bool, "output_LC_Laser_l1"=w1575:bool, "output_LC_Event_l1"=w1576:bool, "output_state"=w1581:T2, "output_dataCurrent"=w1580:u16[], "output_dataTrial"=w1569:u16[][], "output_anySelect_L"=w1571:bool, "output_anySelect_R"=w1572:bool)  [unwired: 2 in]
                  n389 = local write "allReward_L"(w1571) -> ()
                  n390 = local write "allReward_R"(w1572) -> ()
                  n391 = local write "error out"(w1587) -> ()
                }
                frame "SelectReward_pre" {
                  n392 = call "BRig_RT__Case_Exp__State_RewardPre.vi"("input_dataCurrent"=w1611, "input_dataBlock"=w1610, "input_dataTrial"=w1601) -> ("output_T_Reward"=w1597:u16, "output_c_nReward_total_R"=w1606:u16, "output_c_nReward_total_L"=w1607:u16, "output_dataCurrent"=w1604:u16[], "output_dataBlock"=w1609:u16[][], "output_c_nReward_total"=w1605:u16, "output_nReward"=w1608:u16, "output_dataTrial"=w1600:u16[][])  [unwired: 5 in]
                  n393 = local read "FPGA_count2ms"() -> (w1596:dbl)
                  n394 = local write "nRewards_Right"(w1606) -> ()
                  n395 = local write "nRewards_Left"(w1607) -> ()
                  n396 = local write "nRewards_cur"(w1608) -> ()
                  n397 = local write "nRewards_total"(w1605) -> ()
                  n398 = To Double Precision Float(number=w1597) -> (double precision float=w1595:dbl)
                  n399 = Multiply(x=w1596, y=w1595) -> (x*y=w1593:dbl)
                  n400 = Round Toward +Infinity(x=w1593) -> (ceil(x): smallest int >= x=w1594:dbl)
                  n401 = call "BRig_RT_comm_tcp_write_RTwrite__RunState_Trial_selResult.vi"("input_dataTrial"=w1600, "iReward_or_iError"=TRUE, "input_dataCurrent"=w1604) -> ("output_strCmd"=w1602:string)  [unwired: 8 in]
                  n402 = To Unsigned Long Integer(number=w1594) -> (unsigned 32bit integer=w1592:u32)
                  n403 = xnode "Read/Write Control"("FPGA VI Reference In"=w1599, "error in"=w1598, "Solenoid_nTotal_L"=w1592, "Solenoid_nTotal_R"=w1592) -> ()  [unwired: 2 out]
                }
                frame "SelectReward" {
                  n404 = call "BRig_dataCurrent_c_generic.vi"() -> ("output_count_generic"=w1621:i32)  [unwired: 11 in]
                  n405 = call "BRig_RT__Case_Exp__State_Reward.vi"("input_dataCurrent"=w1622, "input_state"=w1626, "input_dataExp"=w1624) -> ("output_state"=w1625:T2, "output_dataCurrent"=w1627:u16[], "output__L"=w1619:bool, "output__R"=w1618:bool)  [unwired: 9 in]
                  n406 = Index Array(array=w1622, index=w1621) -> (element=w1620:u16)
                  n407 = Equal To 0?(x=w1620) -> (x = 0?=w1617:bool)
                  n408 = And(x=w1619, y=w1617) -> (x .and. y?=w1616:bool)
                  n409 = And(x=w1618, y=w1617) -> (x .and. y?=w1615:bool)
                }
                frame "SelectRewardPost_pre" {
                  n410 = call "BRig_dataExp_T_RewardPost.vi"() -> ("output_T_RewardPost"=w1631:i32)  [unwired: 11 in]
                  n411 = call "BRig_dataCurrent_c_generic.vi"() -> ("output_count_generic"=w1637:i32)  [unwired: 11 in]
                  n412 = call "BRig_dataCurrent_T_generic.vi"() -> ("output_T_generic"=w1636:i32)  [unwired: 11 in]
                  n413 = Index Array(array=w1632, index=w1631) -> (element=w1630:u16)
                  n414 = Replace Array Subset(array=w1634, new element #1=u16 0 ("new element/subarray"), index #1=w1637, new element #2=w1630, index #2=w1636) -> (w1633:u16[])
                }
                frame "SelectRewardPost" {
                  n415 = call "BRig_RT__Case_Exp__generic__incrementCountTilThreshold.vi"("input_dataCurrent"=w1644) -> ("output_dataCurrent"=w1642:u16[], "output_underThreshold"=w1643:bool)  [unwired: 9 in]
                  n416 = Select(t=w1646, s=w1643, f=myRIO_BRig_RT__Case_Exp_stateList."endTrial1" ("Enum")) -> (s? t:f=w1645:T2)
                }
                frame "SelectWrong_pre" {
                  n417 = call "BRig_RT__Case_Exp__State_WrongOrTimeout_Pre__v3.vi"("input_dataCurrent"=w1668, "input_WorTO"=FALSE, "input_dataBlock"=w1666, "input_dataTrial"=w1663, "input_dataExp"=w1664) -> ("output_BTPR"=w1657:bool, "output_T2R"=w1658:bool, "output_T2R_or_BTPR"=w1656:u16, "output_dataCurrent"=w1661:u16[], "output_dataBlock"=w1665:u16[][], "output_dataTrial"=w1660:u16[][], "output_BTPRavg"=w1652:dbl, "output_T2Ravg"=w1653:dbl, "output_R(F)_or_L(T)"=w1654:bool, "output_haveNewAvg"=w1655:bool)  [unwired: 1 in]
                  n418 = case shown="True" w1655 {
                    tunnel: w1654 -> [_ w1673]
                    tunnel: w1653 -> [_ w1672]
                    tunnel: w1652 -> [_ w1671]
                    frame False {
                    }
                    frame True {
                      n419 = case shown="False" w1673 {
                        tunnel: w1672 -> [w1674 w1677]
                        tunnel: w1671 -> [w1675 w1676]
                        frame False {
                          n420 = local write "BTPR_avg_R"(w1675) -> ()
                          n421 = local write "T2R_avg_R"(w1674) -> ()
                        }
                        frame True {
                          n422 = local write "BTPR_avg_L"(w1676) -> ()
                          n423 = local write "T2R_avg_L"(w1677) -> ()
                        }
                      }
                    }
                  }
                  n424 = case shown="True" w1658 {
                    tunnel: w1656 -> [_ w1678]
                    frame False {
                    }
                    frame True {
                      n425 = local write "T2R_block"(w1678) -> ()
                    }
                  }
                  n426 = case shown="True" w1657 {
                    tunnel: w1656 -> [_ w1679]
                    frame False {
                    }
                    frame True {
                      n427 = local write "BTPR_block"(w1679) -> ()
                    }
                  }
                  n428 = call "BRig_RT_comm_tcp_write_RTwrite__RunState_Trial_selResult.vi"("input_dataTrial"=w1660, "iReward_or_iError"=FALSE, "input_dataCurrent"=w1661) -> ("output_strCmd"=w1659:string)  [unwired: 8 in]
                }
                frame "SelectWrong" {
                  n429 = call "BRig_RT__Case_Exp__generic__incrementCountTilThreshold.vi"("input_dataCurrent"=w1682) -> ("output_dataCurrent"=w1680:u16[], "output_underThreshold"=w1681:bool)  [unwired: 9 in]
                  n430 = Select(t=w1684, s=w1681, f=myRIO_BRig_RT__Case_Exp_stateList."endTrial1" ("Enum")) -> (s? t:f=w1683:T2)
                }
                frame "SelectTimeout_pre" {
                  n431 = call "BRig_RT__Case_Exp__State_WrongOrTimeout_Pre__v3.vi"("input_dataCurrent"=w1706, "input_WorTO"=TRUE, "input_dataBlock"=w1705, "input_dataTrial"=w1704, "input_dataExp"=w1701) -> ("output_BTPR"=w1695:bool, "output_T2R"=w1696:bool, "output_T2R_or_BTPR"=w1694:u16, "output_dataCurrent"=w1699:u16[], "output_dataBlock"=w1703:u16[][], "output_dataTrial"=w1698:u16[][], "output_BTPRavg"=w1690:dbl, "output_T2Ravg"=w1691:dbl, "output_R(F)_or_L(T)"=w1692:bool, "output_haveNewAvg"=w1693:bool)  [unwired: 1 in]
                  n432 = xnode "Read/Write Control"("FPGA VI Reference In"=w1710, "error in"=w1709, "SelectionState"=FALSE) -> ("error out"=w1707:errorcluster)  [unwired: 1 out]
                  n433 = case shown="True" w1693 {
                    tunnel: w1692 -> [_ w1715]
                    tunnel: w1691 -> [_ w1714]
                    tunnel: w1690 -> [_ w1713]
                    frame False {
                    }
                    frame True {
                      n434 = case shown="False" w1715 {
                        tunnel: w1714 -> [w1716 w1719]
                        tunnel: w1713 -> [w1717 w1718]
                        frame False {
                          n435 = local write "BTPR_avg_R"(w1717) -> ()
                          n436 = local write "T2R_avg_R"(w1716) -> ()
                        }
                        frame True {
                          n437 = local write "BTPR_avg_L"(w1718) -> ()
                          n438 = local write "T2R_avg_L"(w1719) -> ()
                        }
                      }
                    }
                  }
                  n439 = local write "error out"(w1707) -> ()
                  n440 = call "BRig_RT_comm_tcp_write_RTwrite__RunState_Trial_selResult.vi"("input_dataTrial"=w1698, "iReward_or_iError"=FALSE, "input_dataCurrent"=w1699) -> ("output_strCmd"=w1697:string)  [unwired: 8 in]
                  n441 = case shown="True" w1695 {
                    tunnel: w1694 -> [_ w1721]
                    frame False {
                    }
                    frame True {
                      n442 = local write "BTPR_block"(w1721) -> ()
                    }
                  }
                  n443 = case shown="True" w1696 {
                    tunnel: w1694 -> [_ w1720]
                    frame False {
                    }
                    frame True {
                      n444 = local write "T2R_block"(w1720) -> ()
                    }
                  }
                }
                frame "SelectTimeout" {
                  n445 = call "BRig_RT__Case_Exp__generic__incrementCountTilThreshold.vi"("input_dataCurrent"=w1724) -> ("output_dataCurrent"=w1723:u16[], "output_underThreshold"=w1722:bool)  [unwired: 9 in]
                  n446 = Select(t=w1726, s=w1722, f=myRIO_BRig_RT__Case_Exp_stateList."endTrial1" ("Enum")) -> (s? t:f=w1725:T2)
                }
                frame "endTrial1" {
                  n447 = call "BRig_RT_comm_tcp_write_RTwrite__RunState_Trial_end.vi"("input_dataCurrent"=w1739) -> ("output_strCmd"=w1738:string)  [unwired: 10 in]
                  n448 = call "BRig_RT__Case_Exp__State_endTrial__v2.vi"("input_dataBlock"=w1735, "input_timeStamp_start"=w1740, "input_dataTrial"=w1747, "input_dataCurrent"=w1739) -> ("output_BTPRavg"=w1732:dbl, "output_T2Ravg"=w1733:dbl, "output_dataTrial"=w1746:u16[][], "output_dataCurrent"=w1741:u16[], "output_R(F)_or_L(T)"=w1734:bool, "output_runTime"=→"T_ExpRun_min":dbl)  [unwired: 2 in]
                  n449 = xnode "Read/Write Control"("FPGA VI Reference In"=w1743, "error in"=w1742, "SelectionState"=FALSE) -> ("error out"=w1744:errorcluster)  [unwired: 1 out]
                  n450 = case shown="False" w1734 {
                    tunnel: w1733 -> [w1750 w1753]
                    tunnel: w1732 -> [w1751 w1752]
                    frame False {
                      n451 = local write "BTPR_avg_R"(w1751) -> ()
                      n452 = local write "T2R_avg_R"(w1750) -> ()
                    }
                    frame True {
                      n453 = local write "BTPR_avg_L"(w1752) -> ()
                      n454 = local write "T2R_avg_L"(w1753) -> ()
                    }
                  }
                  n455 = local write "error out"(w1744) -> ()
                }
                frame "endTrial2" {
                  n456 = case shown="True" w1763 {
                    tunnel: [w1771 _] -> w1764
                    tunnel: [w1770 w1773] -> w1759
                    tunnel: w1758 -> [w1768 w1781]
                    tunnel: w1757 -> [w1769 w1779]
                    tunnel: [w1769 w1778] -> w1756
                    tunnel: [w1768 w1780] -> w1755
                    tunnel: w1754 -> [_ w1772]
                    frame False {
                      # "Receive commands"
                      n457 = call "BRig_RT__Case_Exp__UploadClosedLoop__v3.vi"() -> ("all rows"=w1771:i64[][], "output_haveCmd"=w1770:bool)  [unwired: 10 in]
                    }
                    frame True {
                      # "Parse commands and update"
                      n458 = Array Size(array=w1772) -> (size(s)=w1777:i32[])
                      n459 = Index Array(array=w1777, index=0) -> (element=w1775:i32)
                      n460 = Not Equal To 0?(x=w1775) -> (x != 0?=w1774:bool)
                      n461 = case shown="False" w1774 {
                        selector: w1774 -> [w1785 w1787]
                        tunnel: w1781 -> [w1783 w1791]
                        tunnel: [w1783 w1790] -> w1780
                        tunnel: w1779 -> [w1782 w1789]
                        tunnel: [w1782 w1788] -> w1778
                        tunnel: [w1785 w1787] -> w1773
                        tunnel: w1772 -> [_ w1786]
                        frame False {
                          w1784 = TRUE ("input_setValues")
                          # "Update"
                          n462 = call "BRig_RT_panel_cue_v0,90.vi"("input_setValues"=w1784, "input_dataExp"=w1783) -> ()  [unwired: 9 in, 1 out]
                          n463 = call "BRig_RT_panel_ExpStruct_v0,96.vi"("input_setValues"=w1784, "input_dataExp"=w1783) -> ()  [unwired: 9 in, 1 out]
                          n464 = call "BRig_RT_panel_Laser1_v0,90.vi"("input_setValues"=w1784, "input_dataExp"=w1783, "input_dataLC"=w1782) -> ()  [unwired: 7 in, 2 out]
                          n465 = call "BRig_RT_panel_Laser2_v0,90.vi"("input_setValues"=w1784, "input_dataExp"=w1783, "input_dataLC"=w1782) -> ()  [unwired: 7 in, 2 out]
                        }
                        frame True {
                          # "Parse"
                          n466 = call "BRig_RT__Case_Exp__UploadClosedLoop__updateSettings.vi"("input_newSettings"=w1786, "input_dataLC"=w1789, "input_dataExp"=w1791) -> ("output_dataLC"=w1788:u16[], "output_dataExp"=w1790:u16[])  [unwired: 7 in]
                        }
                      }
                    }
                  }
                  n467 = Select(t=myRIO_BRig_RT__Case_Exp_stateList."endTrial2", s=w1759, f=myRIO_BRig_RT__Case_Exp_stateList."endTrial3" ("Enum")) -> (s? t:f=w1760:T2)
                }
                frame "endTrial3" {
                  n468 = call "BRig_RT__Case_Exp__endTrial_checkFreeReward.vi"("input_dataBlock"=w1793, "input_dataExp"=w1802, "input_dataTrial"=w1803, "input_dataCurrent"=w1804) -> ("output_state"=w1794:T2, "output_endBlock"=w1792:bool)  [unwired: 6 in]
                  n469 = local read "STOP_endTrial"() -> (w1801:bool)
                  n470 = local read "STOP_abort"() -> (w1800:bool)
                  n471 = local read "START"() -> (w1798:bool)
                  n472 = Not(x=w1798) -> (.not. x?=w1799:bool)
                  n473 = Compound Arithmetic op=OR(w1801, w1799, w1800, w1792) -> (w1797:bool)
                  n474 = Select(t=myRIO_BRig_RT__Case_Exp_stateList."saveData_dataBlock" ("Enum"), s=w1797, f=w1794) -> (s? t:f=w1795:T2)
                }
                frame "endBlock" {
                  # "Get latest\nlaserSwitch"
                  n475 = call "BRig_dataExp_Loop_c_ExpStruct.vi"() -> ("output_Loop_c_ExpStruct"=w1813:i32)  [unwired: 11 in]
                  n476 = call "BRig_dataExp_LaserSwitch.vi"() -> ("output_LaserSwitch"=w1807:i32)  [unwired: 11 in]
                  n477 = local read "START"() -> (w1833:bool)
                  n478 = local read "STOP_endBlock"() -> (w1829:bool)
                  n479 = local read "STOP_endTrial"() -> (w1831:bool)
                  n480 = local read "STOP_abort"() -> (w1830:bool)
                  n481 = Replace Array Subset(array=w1814, new element=u16 2 ("new element/subarray"), index=w1813) -> (w1811:u16[])
                  n482 = call "BRig_RT_panel_ExpStruct_v0,96.vi"("input_setValues"=FALSE, "input_dataExp"=w1811) -> ("output_dataExp"=w1810:u16[])  [unwired: 9 in]
                  n483 = Index Array(array=w1810, index=w1807) -> (element=w1806:u16)
                  n484 = Not(x=w1833) -> (.not. x?=w1832:bool)
                  n485 = Select(t=myRIO_BRig_RT__Case_Exp_stateList."commUpload_dataTrial" ("Enum"), s=w1819, f=myRIO_BRig_RT__Case_Exp_stateList."initBlock" ("Enum")) -> (s? t:f=w1816:T2)
                  n486 = Replace Array Subset(array=w1809, new element=w1806, index=w1807) -> (w1808:u16[])
                  n487 = Compound Arithmetic op=OR(w1832, w1829, w1831, w1830) -> (w1823:bool)
                  n488 = Select(t=myRIO_BRig_RT__Case_Exp_stateList."endExp" ("Enum"), s=w1823, f=w1816) -> (s? t:f=w1834:T2)
                  n489 = Select(t="<S,E>" ("string"), s=w1823, f="") -> (s? t:f=w1820:string)
                }
                frame "endExp" {
                  n490 = xnode "Read/Write Control"("FPGA VI Reference In"=w1837, "error in"=w1836, "A6_Act"=FALSE) -> ("error out"=w1838:errorcluster)  [unwired: 1 out]
                  n491 = local write "error out"(w1838) -> ()
                }
                frame "commUpload_dataTrial" {
                }
                frame "saveData_dataBlock" {
                  n492 = Increment(x=w1868) -> (x+1=w1866:u16)
                  n493 = Replace Array Subset(array=w1860, new element=u16 2 ("new element/subarray"), index=0) -> (w1854:u16[])
                  n494 = Index Array(array=w1852, index (row)=0) -> (element=w1855:u16[])  [unwired: 1 in]
                  n495 = for {
                    tunnel: w1855 -> [w1878] mode=indexing
                    shift-right: [w1877] -> w1853
                    shift-left: w1854 -> [w1881]
                    i -> [w1880]
                    n496 = Increment(x=w1880) -> (x+1=w1879:i32)
                    n497 = Replace Array Subset(array=w1881, new element=w1878, index=w1879) -> (w1877:u16[])
                  }
                  n498 = RT FIFO Write(0:w1863, 1:w1853, 3:w1862) -> (11:w1865:errorcluster)  [unwired: 2 in, 3 out]
                  n499 = Unbundle By Name(w1865) -> ("code"=w1864:i32)
                  n500 = Greater?(x=w1866, y=u16 3) -> (0:w1874:bool)
                  n501 = Equal To 0?(x=w1864) -> (x = 0?=w1861:bool)
                  n502 = Or(x=w1874, y=w1861) -> (x .or. y?=w1873:bool)
                  n503 = Select(t=myRIO_BRig_RT__Case_Exp_stateList."endBlock" ("Enum"), s=w1873, f=w1869) -> (s? t:f=w1867:T2)
                }
                frame "saveData_dataTrial" {
                  n504 = Increment(x=w1899) -> (x+1=w1898:u16)
                  n505 = Replace Array Subset(array=w1884, new element=u16 1 ("new element/subarray"), index=0) -> (w1888:u16[])
                  n506 = Index Array(array=w1883, index (row)=0) -> (element=w1889:u16[])  [unwired: 1 in]
                  n507 = for {
                    tunnel: w1889 -> [w1908] mode=indexing
                    shift-right: [w1907] -> w1887
                    shift-left: w1888 -> [w1911]
                    i -> [w1910]
                    n508 = Increment(x=w1910) -> (x+1=w1909:i32)
                    n509 = Replace Array Subset(array=w1911, new element=w1908, index=w1909) -> (w1907:u16[])
                  }
                  n510 = RT FIFO Write(0:w1886, 1:w1887, 3:w1885) -> (11:w1894:errorcluster)  [unwired: 2 in, 3 out]
                  n511 = Unbundle By Name(w1894) -> ("code"=w1893:i32)
                  n512 = Equal To 0?(x=w1893) -> (x = 0?=w1882:bool)
                  n513 = Greater?(x=w1898, y=u16 3) -> (0:w1896:bool)
                  n514 = Or(x=w1896, y=w1882) -> (x .or. y?=w1895:bool)
                  n515 = Select(t=myRIO_BRig_RT__Case_Exp_stateList."endTrial2" ("Enum"), s=w1895, f=w1900) -> (s? t:f=w1901:T2)
                }
                frame "dummyState" {
                  n516 = call "BRig_dataCurrent_iTrial.vi"() -> ("output_iTrial"=w1918:i32)  [unwired: 11 in]
                  n517 = Index Array(array=w1919, index=w1918) -> (element=w1917:u16)
                  n518 = Equal?(x=w1917, y=u16 1) -> (x = y?=w1915:bool)
                  n519 = Equal To 0?(x=w1926) -> (x = 0?=w1927:bool)
                  n520 = Select(t=u16 13, s=w1915, f=u16 15) -> (s? t:f=w1912:u16)
                  n521 = Select(t=w1912, s=w1927, f=w1926) -> (s? t:f=w1925:u16)
                  n522 = Decrement(x=w1925) -> (x-1=w1924:u16)
                  n523 = Equal To 0?(x=w1924) -> (x = 0?=w1923:bool)
                  n524 = Select(t=myRIO_BRig_RT__Case_Exp_stateList."initTrial" ("Enum"), s=w1923, f=w1921) -> (s? t:f=w1920:T2)
                }
                frame "dummyState_endBlock" {
                  n525 = call "BRig_dataCurrent_iTrial.vi"() -> ("output_iTrial"=w1942:i32)  [unwired: 11 in]
                  n526 = Index Array(array=w1936, index=w1942) -> (element=w1932:u16)
                  n527 = Equal?(x=w1932, y=u16 1) -> (x = y?=w1940:bool)
                  n528 = Equal To 0?(x=w1933) -> (x = 0?=w1944:bool)
                  n529 = Select(t=u16 1, s=w1940, f=u16 3) -> (s? t:f=w1937:u16)
                  n530 = Select(t=w1937, s=w1944, f=w1933) -> (s? t:f=w1943:u16)
                  n531 = Decrement(x=w1943) -> (x-1=w1934:u16)
                  n532 = Equal To 0?(x=w1934) -> (x = 0?=w1935:bool)
                  n533 = Select(t=myRIO_BRig_RT__Case_Exp_stateList."initBlock" ("Enum"), s=w1935, f=w1946) -> (s? t:f=w1945:T2)
                }
                frame "FreeReward_pre" {
                  w1976 = u16 0 ("new element/subarray")
                  # "Duration = MTrig duration"
                  # "Duration = Reward Time"
                  n534 = call "BRig_dataCurrent_FreeReward_c.vi"() -> ("output_FreeReward_c"=w1977:i32)  [unwired: 11 in]
                  n535 = call "BRig_dataCurrent_iSpout.vi"() -> ("output_iSpout"=w1974:i32)  [unwired: 11 in]
                  n536 = call "BRig_dataTrial_T_Reward.vi"() -> ("output_T_Reward"=w1978:i32)  [unwired: 11 in]
                  n537 = call "BRig_dataCurrent_c_generic.vi"() -> ("output_count_generic"=w1983:i32)  [unwired: 11 in]
                  n538 = call "BRig_dataCurrent_T_generic.vi"() -> ("output_T_generic"=w1982:i32)  [unwired: 11 in]
                  n539 = Index Array(array=w1975, index=w1974) -> (element=w1973:u16)
                  n540 = call "BRig_dataMTrig_Solenoid_T_L.vi"() -> ("output_Solenoid_T_L"=w1972:i32)  [unwired: 11 in]
                  n541 = call "BRig_dataMTrig_Solenoid_T_R.vi"() -> ("output_Solenoid_T_R"=w1971:i32)  [unwired: 11 in]
                  n542 = Equal To 0?(x=w1973) -> (x = 0?=w1953:bool)
                  n543 = local read "FPGA_count2ms"() -> (w1965:dbl)
                  n544 = Select(t=w1972, s=w1953, f=w1971) -> (s? t:f=w1969:i32)
                  n545 = Index Array(array=w1979, index (row)=0 ("disabled index (row)"), index (col)=w1978) -> ()  [unwired: 1 out]
                  n546 = Index Array(array=w1970, index=w1969) -> (element=w1964:u16)
                  n547 = Replace Array Subset(array=w1975, new element #1=w1976, index #1=w1977, new element #2=w1976, index #2=w1983, new element #3=w1964, index #3=w1982) -> (w1981:u16[])
                  n548 = To Double Precision Float(number=w1964) -> (double precision float=w1968:dbl)
                  n549 = call "BRig_dataExp_FreeReward_c_L.vi"() -> ("output_FreeReward_c_L"=w1958:i32)  [unwired: 11 in]
                  n550 = call "BRig_dataExp_FreeReward_c_R.vi"() -> ("output_FreeReward_c_R"=w1959:i32)  [unwired: 11 in]
                  n551 = Multiply(x=w1965, y=w1968) -> (x*y=w1966:dbl)
                  n552 = Select(t=w1958, s=w1953, f=w1959) -> (s? t:f=w1955:i32)
                  n553 = Round Toward +Infinity(x=w1966) -> (ceil(x): smallest int >= x=w1967:dbl)
                  n554 = Index Array(array=w1956, index=w1955) -> (element=w1954:u16)
                  n555 = To Unsigned Long Integer(number=w1967) -> (unsigned 32bit integer=w1961:u32)
                  n556 = xnode "Read/Write Control"("FPGA VI Reference In"=w1963, "error in"=w1962, "Solenoid_nTotal_L"=w1961, "Solenoid_nTotal_R"=w1961) -> ()  [unwired: 2 out]
                  n557 = Increment(x=w1954) -> (x+1=w1952:u16)
                  n558 = case shown="False" w1953 {
                    tunnel: w1952 -> [w1986 w1987]
                    frame True {
                      n559 = local write "FreeReward_c_L"(w1986) -> ()
                    }
                    frame False {
                      n560 = local write "FreeReward_c_R"(w1987) -> ()
                    }
                  }
                  n561 = Replace Array Subset(array=w1956, new element=w1952, index=w1955) -> (w1957:u16[])
                }
                frame "FreeReward" {
                  n562 = call "BRig_dataCurrent_iSpout.vi"() -> ("output_iSpout"=w1998:i32)  [unwired: 11 in]
                  n563 = call "BRig_dataCurrent_c_generic.vi"() -> ("output_count_generic"=w1992:i32)  [unwired: 11 in]
                  n564 = Index Array(array=w1999, index #1=w1998, index #2=w1992) -> (element #1=w1997:u16, element #2=w1991:u16)
                  n565 = Equal To 0?(x=w1997) -> (x = 0?=w1995:bool)
                  n566 = Equal To 0?(x=w1991) -> (x = 0?=w1990:bool)
                  n567 = Not(x=w1995) -> (.not. x?=w1996:bool)
                  n568 = call "BRig_RT__Case_Exp__generic__incrementCountTilThreshold.vi"("input_dataCurrent"=w1999) -> ("output_dataCurrent"=w2000:u16[], "output_underThreshold"=w1989:bool)  [unwired: 9 in]
                  n569 = Select(t=w2003, s=w1989, f=myRIO_BRig_RT__Case_Exp_stateList."FreeRewardPost_pre" ("Enum")) -> (s? t:f=w2001:T2)
                  n570 = And(x=w1989, y=w1990) -> (x .and. y?=w1988:bool)
                  n571 = And(x=w1988, y=w1995) -> (x .and. y?=w1993:bool)
                  n572 = And(x=w1988, y=w1996) -> (x .and. y?=w1994:bool)
                }
                frame "FreeRewardPost" {
                  n573 = call "BRig_RT__Case_Exp__generic__incrementCountTilThreshold.vi"("input_dataCurrent"=w2010) -> ("output_dataCurrent"=w2009:u16[], "output_underThreshold"=w2008:bool)  [unwired: 9 in]
                  n574 = Select(t=w2013, s=w2008, f=myRIO_BRig_RT__Case_Exp_stateList."initTrial" ("Enum")) -> (s? t:f=w2011:T2)
                }
                frame "FreeRewardPost_pre" {
                  n575 = call "BRig_dataExp_T_RewardPost.vi"() -> ("output_T_RewardPost"=w2023:i32)  [unwired: 11 in]
                  n576 = call "BRig_dataCurrent_c_generic.vi"() -> ("output_count_generic"=w2026:i32)  [unwired: 11 in]
                  n577 = call "BRig_dataCurrent_T_generic.vi"() -> ("output_T_generic"=w2025:i32)  [unwired: 11 in]
                  n578 = Index Array(array=w2020, index=w2023) -> (element=w2022:u16)
                  n579 = Replace Array Subset(array=w2021, new element #1=u16 0 ("new element/subarray"), index #1=w2026, new element #2=w2022, index #2=w2025) -> (w2019:u16[])
                }
              }
              n580 = call "BRig_RT_panel_manualTriggering_v0,90.vi"("input_dataMTrig"=w1184) -> ("output_Solenoid_R"=w1195:bool, "output_Solenoid_L"=w1194:bool, "output_dataMTrig"=w1227:u16[], "output_Audio_L"=w1226:bool, "output_Audio_R"=w1225:bool, "output_CueLed"=w1223:bool, "output_Laser_l1"=w1199:bool, "output_Laser_l2"=w1219:bool)  [unwired: 11 in]
              n581 = call "BRig_RT__Case_Exp__comm_tcp__data_other.vi"("input_strState"=w1187, "input_strAccum"=w1188, "input_error"=w1189, "input_hTCP"=w1190, "input_I_connected_TCP"=w1191) -> ("output_strAccum"=w1170:string, "output_error"=w1169:errorcluster, "output_hTCP"=w1171:refnum<k5>, "output_I_connect_TCP"=w1172:bool)  [unwired: 3 in]
              n582 = Or(x="STOP_abort", y=w1211) -> (x .or. y?=w1173:bool)
              n583 = Or(x=w1224, y=w1223) -> (x .or. y?=w1202:bool)
              n584 = local read "Laser1_LED"() -> (w1160:bool)
              n585 = local read "Laser2_LED"() -> (w1159:bool)
              n586 = Or(x=w1226, y=w1241) -> (x .or. y?=w1201:bool)
              n587 = Or(x=w1240, y=w1225) -> (x .or. y?=w1200:bool)
              n588 = Or(x=w1198, y=w1199) -> (x .or. y?=w1218:bool)
              n589 = Or(x=w1222, y=w1219) -> (x .or. y?=w1220:bool)
              n590 = call "BRig_RT__Case_Exp__recordLick.vi"("input_dataLick"=w1210, "input_lick__R"=w1204, "input_lick__L"=w1205, "input_lick"=w1206, "intput_state__trialStart"=w1164, "intput_state__trialEnd"=w1209, "input_dataCurrent"=w1208) -> ("output_dataLick"=w1203:u16[][], "output_dataCurrent"=w1207:u16[])  [unwired: 7 in]
              n591 = xnode "Read/Write Control"("FPGA VI Reference In"=w1239, "error in"=w1238, "L1Led_ON"=w1160, "L2Led_ON"=w1159, "Solenoid_trig_L"=w1193, "Solenoid_trig_R"=w1192, "A3_SL"=w1194, "A1_SR"=w1195, "LC_Event_l1"=w1217, "LC_Laser_l1"=w1218, "LC_Event_l2"=w1221, "LC_Laser_l2"=w1220, "CueLed_Event"=w1202, "audioTrigger_L"=w1201, "audioTrigger_R"=w1200) -> ("FPGA VI Reference Out"=w1245:refnum<k20>, "error out"=w1244:errorcluster, "AnaIn_0"=w1185:i16, "AnaIn_1"=w1186:i16)
              n592 = call "BRig_RT__Case_Exp__recordAnalogInput__PortC__fifo__1value.vi"("input_iOccurence"=w1215, "resetOccurrence"=w1214, "input_dataCurrent"=w1208, "input_iState_start"=w1164, "rt fifo"=w1163, "input_iState_end"=w1209, "input_fifo_error"=w1162, "input_AI1"=w1186, "input_AI0"=w1185) -> ("output_fifo_error"=w1168:errorcluster, "output_iOccurrence"=w1216:u16)  [unwired: 8 in, 1 out]
              n593 = call "BRig_RT_timeLoop_Exp__noStateLimit.vi"("input_error"=w1168, "input_Threshold_reset"="input_Threshold_reset", "input_Threshold"=w1230, "input_timestamp"=w1231, "input_state"=w1164) -> ("output_Threshold"=w1228:bool, "output_duration"=→"tLoop":dbl)  [unwired: 4 in, 1 out]
              "Threshold" <- w1228
              n594 = node-c288() -> ()  [unwired: 1 in, 1 out]
            }
            "stop_TimedLoop" <- w861
            n595 = while {
              tunnel: w803 -> [w929]
              tunnel: w802 -> [w928]
              shift-right: [w923] -> _
              shift-left: 0 ("element") -> [w924]
              shift-right: [w919] -> _
              shift-left: w808 -> [w925]
              tunnel: [w922] -> w805
              tunnel: [w921] -> w804
              tunnel: w801 -> [w918]
              tunnel: w800 -> [w917]
              tunnel: [w916] -> w799
              tunnel: [w915] -> w798
              shift-right: [w913] -> _
              shift-left: FALSE -> [w914]
              stop <- w912 stop-if-true
              # "timed out?"
              n596 = RT FIFO Read(0:w929, 3:w928) -> (8:w922:refnum<k33>, 9:w926:u16, 10:w933:bool, 11:w930:errorcluster)  [unwired: 2 in, 1 out]
              n597 = Unbundle By Name(w930) -> ("code"=w934:i32)
              n598 = Not(x=w933) -> (.not. x?=w932:bool)
              n599 = Equal To 0?(x=w934) -> (x = 0?=w931:bool)
              n600 = And(x=w931, y=w932) -> (x .and. y?=w927:bool)
              n601 = Select(t=w930, s=w931, f=w928) -> (s? t:f=w921:errorcluster)
              n602 = case shown="True" w927 {
                tunnel: w926 -> [_ w965]
                tunnel: w925 -> [w957 w967]
                tunnel: w924 -> [w956 w964]
                tunnel: [w957 w966] -> w919
                tunnel: [w956 w960] -> w923
                tunnel: [_ w958] -> w920
                frame False {
                }
                frame True {
                  n603 = Replace Array Subset(array=w967, new element=w965, index=w964) -> (w966:u16[])
                  n604 = Increment(x=w964) -> (x+1=w962:i32)
                  n605 = Less?(x=w964, y=7 ("dimension size")) -> (x < y?=w959:bool)
                  n606 = Select(t=w962, s=w959, f=0) -> (s? t:f=w960:i32)
                  n607 = Not(x=w959) -> (.not. x?=w958:bool)
                }
              }
              n608 = case shown="True" w920 {
                tunnel: w919 -> [_ w946]
                tunnel: w918 -> [w937 w945]
                tunnel: w917 -> [w936 w944]
                tunnel: [w937 w942] -> w916
                tunnel: [w936 w941] -> w915
                tunnel: w914 -> [w935 w939]
                tunnel: [w935 w938] -> w913
                frame False {
                }
                frame True {
                  n609 = for {
                    N: 8 -> [_]
                    tunnel: w946 -> [w953] mode=indexing
                    tunnel: w945 -> [w955]
                    tunnel: w944 -> [w954]
                    shift-right: [w948] -> w940
                    shift-left: FALSE -> [w952]
                    tunnel: [w951] -> w942
                    tunnel: [w950] -> w941
                    n610 = shared-variable-write(w955, w954, w953) -> (w951:refnum<k21>, w950:errorcluster, w949:bool)  [unwired: 1 in]
                    n611 = Or(x=w952, y=w949) -> (x .or. y?=w948:bool)
                  }
                  n612 = Or(x=w939, y=w940) -> (x .or. y?=w938:bool)
                }
              }
              n613 = local read "stop_TimedLoop"() -> (w912:bool)
            }
            n614 = while {
              shift-right: [w1027] -> _
              shift-left: 0 -> [w1016]
              tunnel: w858 -> [w1034]
              tunnel: w850 -> [w1036]
              shift-right: [w1023] -> _
              shift-left: 0 -> [w1018]
              shift-right: [w1028] -> _
              shift-left: w824 -> [w1035]
              shift-right: [w1024] -> _
              shift-left: w823 -> [w1037]
              shift-right: [w1031] -> w847
              shift-left: w817 -> [w1044]
              shift-right: [w1032] -> w840
              shift-left: w816 -> [w1038]
              tunnel: w820 -> [w1021]
              tunnel: w825 -> [w1020]
              stop <- w1045 stop-if-true
              # "nColumns dataBlock"
              # "nColumns dataTrial"
              # "buffer_dataTrial"
              # "buffer_dataBlock"
              # "buffer_dataTrial"
              # "buffer_dataBlock"
              n615 = local read "stop_TimedLoop"() -> (w1045:bool)
              n616 = Not Equal To 0?(x=w1018) -> (x != 0?=w1019:bool)
              n617 = case shown="True" w1019 {
                tunnel: w1037 -> [w1120 w1123]
                tunnel: w1018 -> [w1121 w1125]
                tunnel: w1036 -> [_ w1134]
                tunnel: [w1121 w1122] -> w1025
                tunnel: [w1120 w1123] -> w1026
                frame False {
                }
                frame True {
                  n618 = Array Subset(array=w1123, length (row)=w1125) -> (w1136:u16[][])  [unwired: 3 in]
                  n619 = call "BRig_dataBlock_iBlock.vi"() -> ("output_iBlock"=w1131:i32)  [unwired: 11 in]
                  n620 = Index Array(array=w1123, index (row)=0, index (col)=w1131) -> (element=w1130:u16)
                  n621 = To Double Precision Float(number=w1136) -> (double precision float=w1135:dbl[][])
                  n622 = Not Equal?(x=u16 1, y=w1130) -> (x != y?=w1128:bool)
                  n623 = call-poly <vilib>:"Write To Spreadsheet File.vi"("delimiter (\\t)"="," ("delimiter (\\t)"), "append to file? (new file:F)"=w1128, "2D data"=w1135, "file path (dialog if empty)"=w1134) -> ("new file path (Not A Path if cancelled)"=w1127:path)  [unwired: 4 in]
                  n624 = call <vilib>:"Is Path and Not Empty.vi"("path"=w1127) -> ("Is Path and Not Empty?"=w1126:bool)  [unwired: 4 in]
                  n625 = Select(t=0, s=w1126, f=w1125) -> (s? t:f=w1122:i32)
                }
              }
              n626 = RT FIFO Read(0:w1044, 3:w1038) -> (8:w1031:refnum<k33>, 9:w1022:u16[], 10:w1042:bool, 11:w1039:errorcluster)  [unwired: 2 in, 1 out]
              n627 = Unbundle By Name(w1039) -> ("code"=w1043:i32)
              n628 = Not(x=w1042) -> (.not. x?=w1041:bool)
              n629 = Equal To 0?(x=w1043) -> (x = 0?=w1040:bool)
              n630 = And(x=w1040, y=w1041) -> (x .and. y?=w1033:bool)
              n631 = Select(t=w1039, s=w1040, f=w1038) -> (s? t:f=w1032:errorcluster)
              n632 = Not Equal To 0?(x=w1016) -> (x != 0?=w1017:bool)
              n633 = case shown="True" w1017 {
                tunnel: w1035 -> [w1103 w1106]
                tunnel: w1016 -> [w1104 w1108]
                tunnel: w1034 -> [_ w1117]
                tunnel: [w1104 w1105] -> w1029
                tunnel: [w1103 w1106] -> w1030
                frame False {
                }
                frame True {
                  n634 = Array Subset(array=w1106, length (row)=w1108) -> (w1119:u16[][])  [unwired: 3 in]
                  n635 = call "BRig_dataTrial_nTrial.vi"() -> ("output_nTrial"=w1114:i32)  [unwired: 11 in]
                  n636 = Index Array(array=w1106, index (row)=0, index (col)=w1114) -> (element=w1113:u16)
                  n637 = To Double Precision Float(number=w1119) -> (double precision float=w1118:dbl[][])
                  n638 = Not Equal?(x=u16 1, y=w1113) -> (x != y?=w1111:bool)
                  n639 = call-poly <vilib>:"Write To Spreadsheet File.vi"("delimiter (\\t)"="," ("delimiter (\\t)"), "append to file? (new file:F)"=w1111, "2D data"=w1118, "file path (dialog if empty)"=w1117) -> ("new file path (Not A Path if cancelled)"=w1110:path)  [unwired: 4 in]
                  n640 = call <vilib>:"Is Path and Not Empty.vi"("path"=w1110) -> ("Is Path and Not Empty?"=w1109:bool)  [unwired: 4 in]
                  n641 = Select(t=0, s=w1109, f=w1108) -> (s? t:f=w1105:i32)
                }
              }
              n642 = case shown="True" w1033 {
                tunnel: w1030 -> [w1050 w1060]
                tunnel: w1029 -> [w1049 w1058]
                tunnel: [w1050 w1059] -> w1028
                tunnel: [w1049 w1057] -> w1027
                tunnel: w1026 -> [w1048 w1056]
                tunnel: w1025 -> [w1047 w1054]
                tunnel: [w1048 w1055] -> w1024
                tunnel: [w1047 w1053] -> w1023
                tunnel: w1022 -> [_ w1063]
                tunnel: w1021 -> [_ w1052]
                tunnel: w1020 -> [_ w1051]
                frame False {
                  n643 = Wait (ms)(milliseconds to wait=u32 10) -> ()  [unwired: 1 out]
                }
                frame True {
                  n644 = Index Array(array=w1063, index=0) -> (element=w1061:u16)
                  n645 = Not Equal To 0?(x=w1061) -> (x != 0?=w1062:bool)
                  n646 = case shown="True" w1062 {
                    tunnel: w1063 -> [_ w1079]
                    tunnel: w1061 -> [_ w1082]
                    tunnel: w1060 -> [w1068 w1072]
                    tunnel: [w1068 w1071] -> w1059
                    tunnel: w1058 -> [w1067 w1070]
                    tunnel: [w1067 w1069] -> w1057
                    tunnel: w1056 -> [w1066 w1076]
                    tunnel: [w1066 w1074] -> w1055
                    tunnel: w1054 -> [w1065 w1075]
                    tunnel: [w1065 w1073] -> w1053
                    tunnel: w1052 -> [_ w1078]
                    tunnel: w1051 -> [_ w1077]
                    frame False {
                    }
                    frame True {
                      n647 = Equal?(x=u16 1 ("y"), y=w1082) -> (x = y?=w1080:bool)
                      n648 = case shown="False" w1080 {
                        tunnel: w1079 -> [w1090 w1102]
                        tunnel: w1078 -> [w1088 _]
                        tunnel: w1077 -> [_ w1097]
                        tunnel: w1076 -> [w1092 w1096]
                        tunnel: w1075 -> [w1091 w1098]
                        tunnel: [w1092 w1095] -> w1074
                        tunnel: [w1091 w1094] -> w1073
                        tunnel: w1072 -> [w1087 w1099]
                        tunnel: [w1085 w1099] -> w1071
                        tunnel: w1070 -> [w1084 w1093]
                        tunnel: [w1083 w1093] -> w1069
                        frame True {
                          n649 = Array Subset(array=w1090, index=1, length=w1088) -> (w1086:u16[])
                          n650 = Increment(x=w1084) -> (x+1=w1083:i32)
                          n651 = Replace Array Subset(array=w1087, new element=w1086, index (row)=w1084) -> (w1085:u16[][])  [unwired: 1 in]
                        }
                        frame False {
                          n652 = Array Subset(array=w1102, index=1, length=w1097) -> (w1100:u16[])
                          n653 = Increment(x=w1098) -> (x+1=w1094:i32)
                          n654 = Replace Array Subset(array=w1096, new element=w1100, index (row)=w1098) -> (w1095:u16[][])  [unwired: 1 in]
                        }
                      }
                    }
                  }
                }
              }
            }
            n655 = node-c288(w910) -> ()  [unwired: 1 out]
            n656 = RT FIFO Delete(0:w847, 2:TRUE ("force destroy? (F)"), 3:w840) -> ()  [unwired: 1 out]
            n657 = RT FIFO Delete(0:w805, 2:TRUE ("force destroy? (F)"), 3:w804) -> ()  [unwired: 1 out]
            n658 = flat-sequence {
              tunnel: w881 -> [w1138]
              tunnel: w880 -> [w1141]
              tunnel: w879 -> [w1140]
              tunnel: w878 -> [w1139]
              tunnel: w877 -> [w1143]
              tunnel: w875 -> [_]
              tunnel: w796 -> [w1145]
              tunnel: w845 -> [w1144]
              tunnel: [w1137] -> w856
              tunnel: w840 -> [_]
              tunnel: w874 -> [w1156]
              tunnel: w873 -> [w1155]
              tunnel: w872 -> [w1154]
              tunnel: [w1153] -> w871
              tunnel: [w1152] -> w870
              tunnel: [w1147] -> w866
              tunnel: w856 -> [w1146]
              frame #0 {
                # "Store"
                n659 = call "BRig_RT__Case_Exp__storeData__endExp__v5__p1.vi"("input_dataCurrent"=w1139, "input_dataLC"=w1144, "input_dataExp"=w1145, "input_dataExp_end"=w1140, "input_dataLC_end"=w1141) -> ("output_True"=w1142:bool)  [unwired: 10 in]
                n660 = call "BRig_RT__Case_Exp__storeData__endExp__v5__p2.vi"("input_dataCurrent"=w1139, "input_dataLick"=w1143, "input_True"=w1142, "input_dataMTrig"=w1138) -> ("output_True"=w1137:bool)  [unwired: 11 in]
              }
              frame #1 {
                # "Send"
                n661 = local read "Data Set Prefix"() -> (w1148:string)
                n662 = call "BRig_RT_comm_webdav_upload_all__v3.vi"("input_I_connected_webdav"=w1154, "input_fileName_prefix"=w1148, "input_hSession"=w1155, "input_error"=w1156, "input_True"=w1146) -> ("output_hSession"=w1152:T4, "error out"=w1153:errorcluster, "output_nFilenames"=w1149:i32, "output_arrFilenames"=w1150:string[], "output_uploaded"=w1151:bool[], "output_strCmd"=w1147:string)  [unwired: 5 in]
                n663 = call "BRig_RT_comm_webdav_upload_all_warnUser.vi"("input_n"=w1149, "input_arrFilenames"=w1150, "input_arrUploaded"=w1151) -> ()  [unwired: 9 in]
              }
            }
            n664 = flat-sequence {
              tunnel: w890 -> [w1157]
              tunnel: [w1157] -> w876
              frame #0 {
                w1158 = FALSE ("START")
                n665 = local write "START"(w1158) -> ()
                n666 = local write "STOP_endTrial"(w1158) -> ()
                n667 = local write "STOP_endBlock"(w1158) -> ()
              }
            }
            n668 = xnode "Read/Write Control"("FPGA VI Reference In"=w907, "error in"=w876, "Counts_Reset"=TRUE, "audioTrigger_L"=w893, "audioFreq_L_kHz"=w891, "audioAmp_L"=w892, "audioTrigger_R"=w893, "audioFreq_R_kHz"=w891, "audioAmp_R"=w892, "A3_SL"=w893, "A1_SR"=w893, "A6_Act"=w893) -> ("FPGA VI Reference Out"=w906:refnum<k20>, "error out"=w875:errorcluster)
            n669 = call "BRig_RT__Case_Exp__comm_tcp__data_other.vi"("input_strState"=w866, "input_strAccum"="" ("f"), "input_error"=w867, "input_hTCP"=w868, "input_I_connected_TCP"=w869) -> ("output_error"=w862:errorcluster, "output_hTCP"=w863:refnum<k5>, "output_I_connect_TCP"=w864:bool)  [unwired: 3 in, 1 out]
          }
        }
        n670 = local read "STOP_abort"() -> (w311:bool)
      }
    }
  }
  n671 = flat-sequence {
    tunnel: w89 -> [w2041]
    tunnel: w88 -> [w2043]
    tunnel: w82 -> [w2042]
    tunnel: [w2042] -> w94
    tunnel: [w2041] -> w93
    tunnel: [w2040] -> w92
    tunnel: w67 -> [w2039]
    tunnel: [w2039] -> w91
    tunnel: w68 -> [w2038]
    tunnel: [w2038] -> w90
    tunnel: w75 -> [w2036]
    tunnel: w74 -> [w2035]
    tunnel: w73 -> [w2034]
    tunnel: w69 -> [w2037]
    tunnel: [w2037] -> w87
    tunnel: w86 -> [_]
    tunnel: [w2036] -> w81
    tunnel: [w2035] -> w80
    tunnel: [w2034] -> w79
    tunnel: w94 -> [w2063]
    tunnel: w93 -> [w2062]
    tunnel: w92 -> [w2061]
    tunnel: [w2060] -> _
    tunnel: w91 -> [w2059]
    tunnel: w90 -> [w2058]
    tunnel: w87 -> [w2057]
    tunnel: w81 -> [w2056]
    tunnel: w80 -> [w2055]
    tunnel: w79 -> [w2054]
    frame #0 {
      # "Stop FPGA\nSend QUIT to Host"
      n672 = case shown="True" w2042 {
        tunnel: w2041 -> [_ w2052]
        tunnel: w2043 -> [w2049 w2051]
        tunnel: [w2049 w2050] -> w2040
        frame False {
        }
        frame True {
          n673 = xnode "Read/Write Control"("FPGA VI Reference In"=w2052, "error in"=w2051, "FPGA_Stop"=TRUE) -> ("error out"=w2050:errorcluster)  [unwired: 1 out]
        }
      }
      n674 = case shown="True" w2036 {
        tunnel: w2035 -> [_ w2048]
        tunnel: w2034 -> [_ w2047]
        frame False {
        }
        frame True {
          w2044 = "<S,Q><S,Q><S,Q><S,Q>" ("input_packet")
          n675 = call "BRig_RT_comm_tcp_write_RTwrite.vi"("input_error"=w2047, "input_packet"=w2044, "input_hTCP"=w2048) -> ("output_error"=w2046:errorcluster, "output_hTCP"=w2045:refnum<k5>)  [unwired: 5 in, 2 out]
          n676 = call "BRig_RT_comm_tcp_write_RTwrite.vi"("input_error"=w2046, "input_packet"=w2044, "input_hTCP"=w2045) -> ()  [unwired: 5 in, 4 out]
        }
      }
    }
    frame #1 {
      # "Disconnect FPGA\nDisconnect comm webdav"
      n677 = case shown="True" w2063 {
        tunnel: w2061 -> [w2068 w2071]
        tunnel: w2062 -> [_ w2070]
        tunnel: [w2068 w2069] -> w2060
        frame False {
        }
        frame True {
          n678 = xnode "Close FPGA VI Reference"("FPGA VI Reference In"=w2070, "error in"=w2071) -> ("error out"=w2072:errorcluster)
          n679 = call <vilib>:"Reset myRIO.vi"("error in (no error)"=w2072) -> ("error out"=w2069:errorcluster)  [unwired: 10 in]
        }
      }
      n680 = case shown="True" w2056 {
        tunnel: w2055 -> [_ w2065]
        tunnel: w2054 -> [_ w2064]
        frame False {
        }
        frame True {
          n681 = TCP Close Connection(connection ID=w2065, error in (no error)=w2064) -> ()  [unwired: 1 in, 2 out]
        }
      }
      n682 = case shown="True" w2059 {
        tunnel: w2058 -> [_ w2067]
        tunnel: w2057 -> [_ w2066]
        frame False {
        }
        frame True {
          n683 = call <vilib>:"Close Session.vi"("session handle"=w2067, "error in (no error)"=w2066) -> ()  [unwired: 13 in, 1 out]
        }
      }
    }
  }
  n684 = Flush Stream(8:w6, 11:w7) -> (0:w8:errorcluster, 3:w9:refnum<k21>)  [unwired: 2 in, 1 out]
  n685 = Destroy Stream Endpoint(8:w8, 11:w9) -> ()  [unwired: 1 out]
